vi "Test.vi"() -> ()   [LabVIEW 2010]
uses:
  Instance           5 12Saved   Test .vi
panel:
  out "Output ALG Msg Last Iter":string[][](table)=[["CODE", "PARAM"]]
  out "Output VOC Msg Last Iter":string[][](table)=[["CODE", "PARAM"]]
  out "Curr step ALG msg counter":i32
  out "Curr step VOC MSG counter":i32
  out "Params":string[](array[string])
  in  "STEP SIZE":i32(knob)=1 scale=1.0..10.0
  in  "Mode":bool
  in  "stop 2":bool
  in  "run":bool
  out "Result Input FOR VOC":u8[](array[numeric])
  out "output array":cluster{i32, "Value":string, i32}[](array[cluster])
  in  "Numeric":u8
  in  "Tab Control":T1(tab)=enum."Output ALG Info"
  out "ALG MSG queue":u8(slide) scale=0.0..5.0
  in  "send msg":bool
  in  "ALG MSG  PARAM":string
  in  "ALG MSG TYPE":string(combo)="0"
  in  "ALG MSG  CODE":string(combo)="1"
  out "VOC MSG queue":u8(slide) scale=0.0..5.0
  in  "send voc msg 2":bool
  in  "VOC MSG  PARAM":string
  in  "VOC MSG TYPE":string(combo)="0"
  in  "VOC MSG  CODE":string(combo)
  in  "VOC Last Interation MSG":i32(listbox)
  in  "VOC Param type":string(combo)
  out "Output Alg Ports":bool[](array[boolean])
  out "Output VOC Msg LOG":string[][](table)=[["CODE", "PARAM"]]
  out "VOC States":string[][](table)
  in  "ALG Param type":string(combo)
  in  "ALG Last Interation MSG":i32(listbox)
  out "Alg States":string[][](table)
  out "Input Alg Ports":bool[](array[boolean])
  out "Output Alg Msg":string[][](table)=[["CODE", "PARAM"]]
  in  "Save as new test":bool
  in  "Save changes in current test":bool
  in  "TEST":string="script_port: 8 /*index*/, 0 /* СЦЕНАРИЙ_ЛОГ_ВХОД_ПИТ_ВЕНТИЛЯТОРА*/ \r\nscript_port: 9 /*index*/, 0 /* СЦЕНАРИЙ_ЛОГ_ВХОД_ПИТ_РЕГ_Т*/ \r\nscript_port: 10 /*index*/, 0 /* СЦЕНАРИЙ_ЛОГ_ВХОД_НАС_ОХЛ*/ \r\nscript_port: 11 /*index*/, 0 /* СЦЕНАРИЙ_ЛОГ_ВХОД_ВАК_НАСОСА*/ \r\nscript_port: 12 /*index*/, 0 /* СЦЕНАРИЙ_ЛОГ_ВХОД_ЗАТВОР_ВАК*/ \r\nscript_port: 13 /*index*/, 0 /* СЦЕНАРИЙ_ЛОГ_ВХОД_САПУН*/ \r\nscript_port: 14 /*index*/, 0 /* СЦЕНАРИЙ_ЛОГ_ВХОД_УСТР_ПЛАВ_ПУСКА*/ \r\nscript_port: 15 /*index*/, 0 /* СЦЕНАРИЙ_ЛОГ_ВХОД_РЕГ_УР*/ \r\nscript_port: 16 /*index*/, 0 /* СЦЕНАРИЙ_ЛОГ_ВХОД_КОМПРЕССОР*/ \r\n\n\n\n\n\n\n\n"
  in  "Tests List":i32(listbox)
  out "voc code":i32[](array[numeric])=[-1, -1, -1, -1, -1, -1, -1, -1, -1, -1, -1, -1, -1, -1, -1, -1, -1, -1, -1, -1, -1, -1, -1, -1, -1, -1, -1, -1, -1, -1, -1, -1, -1, -1, -1, -1, -1, -1, -1, -1, -1, -1, -1, -1, -1, -1, -1, -1, -1, -1, -1, -1, -1, -1, -1, -1, -1, -1, -1, -1, -1, -1, -1, -1, -1, -1, -1, -1, -1, -1, -1, -1, -1, -1, -1, -1, -1, -1, -1, -1, -1, -1, -1, -1, -1, -1, -1, -1, -1, -1, -1, -1, -1, -1, -1, -1, -1, -1, -1, -1, -1, -1, -1, -1, -1, -1, -1, -1, -1, -1, -1, -1, -1, -1, -1, -1, -1, -1, -1, -1, -1, -1, -1, -1, -1, -1, -1, -1, -1, -1, -1, -1, -1, -1, -1, -1, -1, -1, -1, -1, -1, -1, -1, -1, -1, -1, -1, -1, -1, -1, -1, -1, -1, -1, -1, -1, -1, -1, -1, -1, -1, -1, -1, -1, -1, -1, -1, -1, -1, -1, -1, -1, -1, -1, -1, -1, -1, -1, -1, -1, -1, -1, -1, -1, -1, -1, -1, -1, -1, -1, -1, -1, -1, -1, -1, -1, -1, -1, -1, -1, -1, -1, -1, -1, -1, -1, -1, -1, -1, -1, -1, -1, -1, -1, -1, -1, -1, -1, -1, -1, -1, -1, -1, -1, -1, -1, -1, -1, -1, -1, -1, -1, -1, -1, -1, -1, -1, -1, -1, -1, -1, -1, -1, -1, -1, -1, -1, -1, -1, -1]
  out "VOC Out MSG Codes":string[](array[string])=["4", "5", "6", "7", "8", "9", "10", "11", "12", "13", "14", "15", "16", "17", "18", "19", "20", "21", "22", "23", "24", "25", "26", "27", "28", "29", "30", "31", "32", "33"]
  out "VOC Out MSG Names":string[](array[string])=["ПК_ТЕСТ_ГУИ_ОШИБКА_КОДА_КОМАНДЫ_ОТ_ГУИ", "ПК_ТЕСТ_ГУИ_ТЕМПЕРАТУРА_ВОДЫ_В_БАКЕ_ИЗМЕНИЛАСЬ", "ПК_ТЕСТ_ГУИ_ТЕМПЕРАТУРА_ВОДЫ_В_РУБАШКЕ_ИЗМЕНИЛАСЬ", "ПК_ТЕСТ_ГУИ_ТЕМПЕРАТУРА_НАСОСА_ИЗМЕНИЛАСЬ", "ПК_ТЕСТ_ГУИ_ВОДА_В_БАКЕ_ЗАКИПЕЛА", "ПК_ТЕСТ_ГУИ_ВОДА_В_БАКЕ_ЗАМЕРЗЛА", "ПК_ТЕСТ_ГУИ_ТЕМПЕРАТУРА_ВОДЫ_В_БАКЕ_СЛИШКОМ_ВЫСОКАЯ", "ПК_ТЕСТ_ГУИ_ТЕМПЕРАТУРА_ВОДЫ_В_БАКЕ_СЛИШКОМ_НИЗКАЯ", "ПК_ТЕСТ_ГУИ_ТЕМПЕРАТУРА_ОКУЖАЮЩЕЙ_СРЕДЫ_ИЗМЕНИЛАСЬ", "ПК_ТЕСТ_ГУИ_ТЕМПЕРАТУРА_ОКУЖАЮЩЕЙ_СРЕДЫ_СЛИШКОМ_ВЫСОКАЯ", "ПК_ТЕСТ_ГУИ_ТЕМПЕРАТУРА_ОКУЖАЮЩЕЙ_СРЕДЫ_СЛИШКОМ_НИЗКАЯ", "ПК_ТЕСТ_ГУИ_УРОВЕНЬ_ВОДЫ_НОРМ", "ПК_ТЕСТ_ГУИ_УРОВЕНЬ_ВОДЫ_MAX", "ПК_ТЕСТ_ГУИ_УРОВЕНЬ_ВОДЫ_MIN", "ПК_ТЕСТ_ГУИ_ДАВЛЕНИЕ_В_ТРУБЕ_СИДЕРОСТАТА_ИЗМЕНИЛОСЬ", "ПК_ТЕСТ_ГУИ_ДАВЛЕНИЕ_В_ТРУБЕ_СЛИШКОМ_ВЫСОКОЕ", "ПК_ТЕСТ_ГУИ_ДАВЛЕНИЕ_В_ТРУБЕ_СЛИШКОМ_НИЗКОЕ", "ПК_ТЕСТ_ГУИ_ДАВЛЕНИЕ_В_ПАТРУБКЕ_ИЗМЕНИЛОСЬ", "ПК_ТЕСТ_ГУИ_ДАВЛЕНИЕ_В_ПАТРУБКЕ_СЛИШКОМ_ВЫСОКОЕ", "ПК_ТЕСТ_ГУИ_ДАВЛЕНИЕ_В_ПАТРУБКЕ_СЛИШКОМ_НИЗКОЕ", "ПК_ТЕСТ_ГУИ_ДАВЛЕНИЕ_В_БАКЕ_КОМПРЕССОРА_ИЗМЕНИЛОСЬ", "ПК_ТЕСТ_ГУИ_ДАВЛЕНИЕ_В_КОМПРЕССОРЕ_СЛИШКОМ_НИЗКОЕ", "ПК_ТЕСТ_ГУИ_ОШИБКА_ПОПЫТКА_ОТКРЫТЬ_САПУН_ПРИ_ОТКРЫТОМ_ЗАТВОРЕ", "ПК_ТЕСТ_ГУИ_ОШИБКА_ПОПЫТКА_ОТКРЫТЬ_ЗАТВОР_ПРИ_ОТКРЫТОМ_САПУНЕ", "ПК_ТЕСТ_ГУИ_ОШИБКА_ДАВЛЕНИЕ_ПАТРУБКА_ВЫШЕ_ДАВЛЕНИЯ_ТРУБЫ", "ПК_ТЕСТ_ГУИ_ОШИБКА_ВКЛЮЧЕНИЕ_НАГРЕВА_ПРИ_НИЗКОМ_УРОВНЕ_ВОДЫ", "ПК_ТЕСТ_ГУИ_ПОПЫТКА_ЗАПУСКА_УСТР_ПЛАВ_ПУСКА_БЕЗ_ПИТАНИЯ", "ПК_ТЕСТ_ГУИ_ОШИБКА_ВКЛЮЧЕНИЕ_НАСОСА_ОХЛ_ПРИ_НИЗКОМ_УРОВНЕ_ВОДЫ", "ПК_ТЕСТ_ГУИ_ОШИБКА_ПЕРЕГРЕВ_ВАК_НАСОСА", "ПК_ТЕСТ_ГУИ_ОШИБКА_ОТКЛЮЧЕНИЕ_ПИТАНИЯ_ВКН_ПРИ_ЗАПУЩЕННОМ_ВКН"]
  out "output VOC array":cluster{i32, "Value":string, i32}[](array[cluster])=[{-1, "Value"="", 0}, {-1, "Value"="", 0}, {-1, "Value"="", 0}, {-1, "Value"="", 0}, {-1, "Value"="", 0}, {-1, "Value"="", 0}, {-1, "Value"="", 0}, {-1, "Value"="", 0}, {-1, "Value"="", 0}, {-1, "Value"="", 0}, {-1, "Value"="", 0}, {-1, "Value"="", 0}, {-1, "Value"="", 0}, {-1, "Value"="", 0}, {-1, "Value"="", 0}]
  out "input VOC array":cluster{i32, "Value":string, i32}[](array[cluster])
  out "AY states array":cluster{u32, u8}[](array[cluster])
  out "ALG output array":cluster{i32, "Value":string, i32}[](array[cluster])=[{-1, "Value"="", 0}, {-1, "Value"="", 0}, {-1, "Value"="", 0}, {-1, "Value"="", 0}, {-1, "Value"="", 0}]
  out "voc states array":cluster{u32, u8}[](array[cluster])
  out "ALG input array":cluster{i32, "Value":string, i32}[](array[cluster])
  out "VOC_STATES_SET":string[][](array[string])=[["Начало", " ", " ", " ", " ", " "], ["Начало", "НекорректноеСобытие", " ", " ", " ", " "], ["Начало", " ", " ", " ", " ", " "], ["Останов", " ", " ", " ", " ", " "], ["Начало", "Неисправность_вентилятора", " ", " ", " ", " "], ["Включение", "Вентилятор_ВКЛЮЧЕН", " ", " ", " ", " "], ["Выключение", "Вентилятор_ВЫКЛЮЧЕН", " ", " ", " ", " "], ["Начало", "Неисправность_Регулятора_Температуры", " ", " ", " ", " "], ["Включение", "Контроль_температуры_ВКЛЮЧЕН", "Временное_Отключение", "Кипение", " ", " "], ["Включение", "Контроль_температуры_ВЫКЛЮЧЕН", "СамопроизвольноеОхлаждение", "СамопроивольныйНагрев", "Замерзло", "ТепловоеРавновесие"], ["Начало", "Неисправность_регулятора_уровня", " ", " ", " ", " "], ["Включение", "Контроль_Рег_Уровня_ВКЛЮЧЕН", " ", " ", " ", " "], ["Включение", "Контроль_Рег_Уровня_ВЫКЛЮЧЕН", " ", " ", " ", " "], ["Начало", "Неисправность_Насоса_Охлаждения", " ", " ", " ", " "], ["Включение", "Контроль_Насоса_Охлажд_ВКЛЮЧЕН", "НАГРЕВ_НАСОСА_ОХЛАЖД_ВОДЫ", "ОХЛАЖД_НАСОСА_НАГРЕВ_ВОДЫ", "ТепловоеРавновесие", "Авария"], ["Включение", "Контроль_Насоса_Охлажд_ВЫКЛЮЧЕН", "САМОПРОИЗВ_ОХЛАЖД_НАСОСА", "САМОПРОИЗВ_НАГРЕВ_НАСОСА", "ТепловоеРавновесие", " "], ["Начало", "Неисправность_Сапуна", " ", " ", " ", " "], ["Открытие", "Сапун_ОТКРЫТ", " ", " ", " ", " "], ["Выключение", "Сапун_ЗАКРЫТ", " ", " ", " ", " "], ["Начало", "Неисправность_Затвора", " ", " ", " ", " "], ["Открытие", "Затвор_ОТКРЫТ", " ", " ", " ", " "], ["Закрытие", "Затвор_ЗАКРЫТ", " ", " ", " ", " "], ["Начало", "Неисправность_питания_насоса", " ", " ", " ", " "], ["Включение", "Питание_ПОДАНО", " ", " ", " ", " "], ["Выключение", "Задержка_перед_отключением", "Питание_ОТКЛЮЧЕНО", " ", " ", " "], ["Начало", "Неисправность_устр_плав_пуска", " ", " ", " ", " "], ["Включение", "Устр_Плав_Пуска_ЗАПУЩЕНО", "Вакуум", " ", " ", " "], ["Выключение", "Устр_Плав_Пуска_ОСТАНОВЛЕНО", " ", " ", " ", " "], ["Начало", "Исправность_Компрессора", "Неисправность_Компрессора", " ", " ", " "]]
  out "VOC_PROC":string[](array[string])=["Инициализация", "ЧтениеКольцевогоБуфера", "ЗАПОЛНЕНИЕ_ДОСТОВЕРНОСТЕЙ", "АварийноеЗавершениеРаботы", "УПРАВЛЕНИЕ_ВЕНТИЛЯТОРОМ", "ВКЛЮЧЕНИЕ_ВЕНТИЛЯТОРА", "ВЫКЛЮЧЕНИЕ_ВЕНТИЛЯТОРА", "УПРАВЛЕНИЕ_ТЕМПЕРАТУРОЙ", "ВКЛЮЧЕНИЕ_РЕГ_ТЕМПЕРАТУРЫ", "ВЫКЛЮЧЕНИЕ_РЕГ_ТЕМПЕРАТУРЫ", "УПРАВЛЕНИЕ_РЕГУЛЯТОРОМ_УР_ВОДЫ_В_БАКЕ", "ВКЛЮЧЕНИЕ_РЕГ_УРОВНЯ", "ВЫКЛЮЧЕНИЕ_РЕГ_УРОВНЯ", "УПРАВЛЕНИЕ_НАСОСОМ_ОХЛАЖДЕНИЯ", "ВКЛЮЧЕНИЕ_НАСОСА_ОХЛАЖД", "ВЫКЛЮЧЕНИЕ_НАСОСА_ОХЛАЖД", "УПРАВЛЕНИЕ_САПУНОМ", "ОТКРЫТИЕ_САПУНА", "ЗАКРЫТИЕ_САПУНА", "УПРАВЛЕНИЕ_ЗАТВОРОМ", "ОТКРЫТИЕ_ЗАТВОРА", "ЗАКРЫТИЕ_ЗАТВОРА", "УПРАВЛЕНИЕ_ПИТАНИЕМ_ВКН", "ПОДАЧА_ПИТАНИЯ_НА_ВКН", "ОТКЛЮЧЕНИЕ_ПИТАНИЯ_ВКН", "УПРАВЛЕНИЕ_УСТР_ПЛАВ_ПУСКА", "ЗАПУСК_УСТР_ПЛАВ_ПУСКА", "ОСТАНОВ_УСТР_ПЛАВ_ПУСКА", "УПРАВЛЕНИЕ_КОМПРЕССОРОМ"]
  out "Alg Out MSG Codes":string[](array[string])=["0", "1", "2", "3", "4", "5", "6", "7", "8", "9", "10", "11", "12", "13", "14", "15", "16", "41", "42", "43", "44", "45", "46", "47", "48", "49", "50", "51", "52", "53", "54", "55", "56", "57", "58", "59", "60", "61", "62", "63", "64", "65", "66", "67", "68", "69", "70", "71", "72", "73", "74", "75", "76", "77", "78", "79", "80", "81", "82", "83", "84", "85", "86", "87", "88", "89", "90", "91", "92", "93", "94", "95", "96", "97", "98", "99", "100", "101", "102", "103", "104", "105", "106", "107", "108", "109", "110", "111", "112", "113", "114", "115", "116", "117", "118", "119", "120", "121", "122", "123", "124", "125", "126", "127", "128", "129", "130", "135"]
  out "Alg Out MSG Names":string[](array[string])=["ПК_ГУИ_УРОВЕНЬ_ВОДЫ_В_БАКЕ_ОХЛАЖДЕНИЯ_НИЗКИЙ", "ПК_ГУИ_УРОВЕНЬ_ВОДЫ_В_БАКЕ_ОХЛАЖДЕНИЯ_ВЫСОКИЙ", "ПК_ГУИ_УРОВЕНЬ_ВОДЫ_В_БАКЕ_ОХЛАЖДЕНИЯ_В_НОРМЕ", "ПК_ГУИ_ОТКАЗ_ДАТЧИКОВ_УРОВНЯ", "ПК_ГУИ_ТЕМПЕРАТУРА_ВОДЫ_В_БАКЕ_ОХЛАЖДЕНИЯ_НИЗКАЯ", "ПК_ГУИ_ТЕМПЕРАТУРА_ВОДЫ_В_БАКЕ_ОХЛАЖДЕНИЯ_ВЫСОКАЯ", "ПК_ГУИ_ТЕМПЕРАТУРА_ВОДЫ_В_БАКЕ_ОХЛАЖДЕНИЯ_В_НОРМЕ", "ПК_ГУИ_ТЕМПЕРАТУРА_ВОДЫ_В_РУБАШКЕ_ОХЛАЖДЕНИЯ_НИЗКАЯ", "ПК_ГУИ_ТЕМПЕРАТУРА_ВОДЫ_В_РУБАШКЕ_ОХЛАЖДЕНИЯ_ВЫСОКАЯ", "ПК_ГУИ_ТЕМПЕРАТУРА_ВОДЫ_В_РУБАШКЕ_ОХЛАЖДЕНИЯ_В_НОРМЕ", "ПК_ГУИ_ДАВЛЕНИЕ_В_ВАКУУМНОЙ_ТРУБЕ_В_НОРМЕ", "ПК_ГУИ_ДАВЛЕНИЕ_В_ВАКУУМНОЙ_ТРУБЕ_ВНЕ_НОРМЫ", "ПК_ГУИ_СКОРОСТЬ_ОТКАЧКИ_В_НОРМЕ", "ПК_ГУИ_СКОРОСТЬ_ОТКАЧКИ_НИЖЕ_НОРМЫ", "ПК_ГУИ_ДАВЛЕНИЕ_В_БАКЕ_КОМПРЕССОРА_В_НОРМЕ", "ПК_ГУИ_ДАВЛЕНИЕ_В_БАКЕ_КОМПРЕССОРА_ВЫШЕ_НОРМЫ", "ПК_ГУИ_ДАВЛЕНИЕ_В_БАКЕ_КОМПРЕССОРА_НИЖЕ_НОРМЫ", "ПК_ГУИ_ОТКАЗ_ОТКРЫТИЯ_ЗАТВОРА_ВАКУУМНОГО", "ПК_ГУИ_ОТКАЗ_ЗАКРЫТИЯ_ЗАТВОРА_ВАКУУМНОГО", "ПК_ГУИ_ОТКАЗ_ОТКРЫТИЯ_САПУНА", "ПК_ГУИ_ОТКАЗ_ЗАКРЫТИЯ_САПУНА", "ПК_ГУИ_ОТКАЗ_ВКЛЮЧЕНИЯ_ВЕНТИЛЯТОРА", "ПК_ГУИ_ОТКАЗ_ВЫКЛЮЧЕНИЯ_ВЕНТИЛЯТОРА", "ПК_ГУИ_ОТКАЗ_ВКЛЮЧЕНИЯ_УСТР_ПЛАВ_ПУСКА", "ПК_ГУИ_ОТКАЗ_ВЫКЛЮЧЕНИЯ_УСТР_ПЛАВ_ПУСКА", "ПК_ГУИ_ОТКАЗ_ВКЛЮЧЕНИЯ_РЕГУЛЯТОРА_ТЕМПЕРАТУРЫ", "ПК_ГУИ_ОТКАЗ_ВЫКЛЮЧЕНИЯ_РЕГУЛЯТОРА_ТЕМПЕРАТУРЫ", "ПК_ГУИ_ОТКАЗ_ВКЛЮЧЕНИЯ_РЕГУЛЯТОРА_УРОВНЯ", "ПК_ГУИ_ОТКАЗ_ВЫКЛЮЧЕНИЯ_РЕГУЛЯТОРА_УРОВНЯ", "ПК_ГУИ_ОТКАЗ_ВКЛЮЧЕНИЯ_НАСОСА_ОХЛАЖДЕНИЯ", "ПК_ГУИ_ОТКАЗ_ВЫКЛЮЧЕНИЯ_НАСОСА_ОХЛАЖДЕНИЯ", "ПК_ГУИ_ИДЕТ_ВАКУУМИРОВАНИЕ_ОТКАЗ_ВЫПОЛНЕНИЯ_КОМАНДЫ", "ПК_ГУИ_НЕТ_УСЛОВИЙ_ДЛЯ_ВЫПОЛНЕНИЯ_КОМАНДЫ", "ПК_ГУИ_УРОВЕНЬ_ВОДЫ_В_БАКЕ_ОХЛАЖДЕНИЯ_ВНЕ_НОРМЫ_ОТКАЗ_ВЫПОЛНЕНИ", "ПК_ГУИ_ОТРИЦАТЕЛЬНАЯ_ТЕМПЕРАТУРА_ВОДЫ_ОТКАЗ_ВЫПОЛНЕНИЯ_КОМАНДЫ", "ПК_ГУИ_ДАВЛЕНИЕ_В_ПАТРУБКЕ_НЕ_УМЕНЬШАЕТСЯ", "ПК_ГУИ_ДАВЛЕНИЕ_В_ВАК_ТРУБЕ_НЕ_УМЕНЬШАЕТСЯ", "ПК_ГУИ_ВАКУУМИРОВАНИЕ_УСПЕШНО_ЗАВЕРШЕНО", "ПК_ГУИ_ОТКАЗ_ВКЛЮЧЕНИЯ_ПИТАНИЯ_ВАКУУМНОГО_НАСОСА", "ПК_ГУИ_ОТКАЗ_ВЫКЛЮЧЕНИЯ_ПИТАНИЯ_ВАКУУМНОГО_НАСОСА", "ПК_ГУИ_АВАРИЯ_НЕДОСТОВЕРНЫЕ_ДАННЫЕ_ОБОРУДОВАНИЯ_ВАК_СИСТЕМЫ", "ПК_ГУИ_ВЕНТИЛЯТОР_ВКЛЮЧЕН", "ПК_ГУИ_ВЕНТИЛЯТОР_ВЫКЛЮЧЕН", "ПК_ГУИ_СПОНТАННОЕ_ВЫКЛЮЧЕНИЕ_ВЕНТИЛЯТОРА", "ПК_ГУИ_СПОНТАННОЕ_ВКЛЮЧЕНИЕ_ВЕНТИЛЯТОРА", "ПК_ГУИ_ЗАТВОР_ВАКУУМНЫЙ_ОТКРЫТ", "ПК_ГУИ_ЗАТВОР_ВАКУУМНЫЙ_ЗАКРЫТ", "ПК_ГУИ_СРЕДНЕЕ_СОСТОЯНИЕ_ЗАТВОРА_ВАКУУМНОГО", "ПК_ГУИ_СОСТОЯНИЕ_ОШИБКИ_ЗАТВОРА_ВАКУУМНОГО", "ПК_ГУИ_СПОНТАННОЕ_ОТКРЫТИЕ_ЗАТ_ВАКУУМНОГО", "ПК_ГУИ_СПОНТАННОЕ_ЗАКРЫТИЕ_ЗАТ_ВАКУУМНОГО", "ПК_ГУИ_САПУН_ОТКРЫТ", "ПК_ГУИ_САПУН_ЗАКРЫТ", "ПК_ГУИ_СПОНТАННОЕ_ОТКРЫТИЕ_САПУНА", "ПК_ГУИ_СПОНТАННОЕ_ЗАКРЫТИЕ_САПУНА", "ПК_ГУИ_ПИТАНИЕ_ВАКУУМНОГО_НАСОСА_ВКЛЮЧЕНО", "ПК_ГУИ_ПИТАНИЕ_ВАКУУМНОГО_НАСОСА_ВЫКЛЮЧЕНО", "ПК_ГУИ_СПОНТАННОЕ_ВКЛЮЧЕНИЕ_ВАКУУМНОГО_НАСОСА", "ПК_ГУИ_СПОНТАННОЕ_ВЫКЛЮЧЕНИЕ_ВАКУУМНОГО_НАСОСА", "ПК_ГУИ_ПИТАНИЕ_РЕГУЛЯТОРА_ТЕМПЕРАТУРЫ_ВКЛЮЧЕНО", "ПК_ГУИ_ПИТАНИЕ_РЕГУЛЯТОРА_ТЕМПЕРАТУРЫ_ВЫКЛЮЧЕНО", "ПК_ГУИ_СПОНТАННОЕ_ВКЛЮЧЕНИЕ_РЕГУЛЯТОРА_ТЕМПЕРАТУРЫ", "ПК_ГУИ_СПОНТАННОЕ_ВЫКЛЮЧЕНИЕ_РЕГУЛЯТОРА_ТЕМПЕРАТУРЫ", "ПК_ГУИ_ПИТАНИЕ_РЕГУЛЯТОРА_УРОВНЯ_ВКЛЮЧЕНО", "ПК_ГУИ_ПИТАНИЕ_РЕГУЛЯТОРА_УРОВНЯ_ВЫКЛЮЧЕНО", "ПК_ГУИ_СПОНТАННОЕ_ВКЛЮЧЕНИЕ_РЕГУЛЯТОРА_УРОВНЯ", "ПК_ГУИ_СПОНТАННОЕ_ВЫКЛЮЧЕНИЕ_РЕГУЛЯТОРА_УРОВНЯ", "ПК_ГУИ_ПИТАНИЕ_НАСОСА_ОХЛАЖДЕНИЯ_ВКЛЮЧЕНО", "ПК_ГУИ_ПИТАНИЕ_НАСОСА_ОХЛАЖДЕНИЯ_ВЫКЛЮЧЕНО", "ПК_ГУИ_СПОНТАННОЕ_ВКЛЮЧЕНИЕ_НАСОСА_ОХЛАЖДЕНИЯ", "ПК_ГУИ_СПОНТАННОЕ_ВЫКЛЮЧЕНИЕ_НАСОСА_ОХЛАЖДЕНИЯ", "ПК_ГУИ_УСТРОЙСТВО_ПЛАВНОГО_ПУСКА_ВКЛЮЧЕНО", "ПК_ГУИ_УСТРОЙСТВО_ПЛАВНОГО_ПУСКА_ВЫКЛЮЧЕНО", "ПК_ГУИ_СПОНТАННОЕ_ВКЛЮЧЕНИЕ_УСТРОЙСТВА_ПЛАВНОГО_ПУСКА", "ПК_ГУИ_СПОНТАННОЕ_ВЫКЛЮЧЕНИЕ_УСТРОЙСТВА_ПЛАВНОГО_ПУСКА", "ПК_ГУИ_ОТКАЗ_ВАКУУМИРОВАНИЯ", "ПК_ГУИ_ОТКАЗ_ВКЛЮЧЕНИЯ_ВАКУУМНОЙ_ПОДСИСТЕМЫ", "ПК_ГУИ_ОТКАЗ_ВЫКЛЮЧЕНИЯ_ВАКУУМНОЙ_ПОДСИСТЕМЫ", "ПК_ГУИ_ЕСТЬ_ДОСТОВЕРНОСТЬ_КОНТРОЛЯ_ОТКРЫТИЯ_ЗАТВОРА_ВАКУУМНОГО", "ПК_ГУИ_НЕТ_ДОСТОВЕРНОСТИ_КОНТРОЛЯ_ОТКРЫТИЯ_ЗАТВОРА_ВАКУУМНОГО", "ПК_ГУИ_ЕСТЬ_ДОСТОВЕРНОСТЬ_КОНТРОЛЯ_ЗАКРЫТИЯ_ЗАТВОРА_ВАКУУМНОГО", "ПК_ГУИ_НЕТ_ДОСТОВЕРНОСТИ_КОНТРОЛЯ_ЗАКРЫТИЯ_ЗАТВОРА_ВАКУУМНОГО", "ПК_ГУИ_ЕСТЬ_ДОСТОВЕРНОСТЬ_КОНТРОЛЯ_САПУНА", "ПК_ГУИ_НЕТ_ДОСТОВЕРНОСТИ_КОНТРОЛЯ_САПУНА", "ПК_ГУИ_ЕСТЬ_ДОСТОВЕРНОСТЬ_КОНТРОЛЯ_УСТР_ПЛАВ_ПУСКА", "ПК_ГУИ_НЕТ_ДОСТОВЕРНОСТИ_КОНТРОЛЯ_УСТР_ПЛАВ_ПУСКА", "ПК_ГУИ_ЕСТЬ_ДОСТОВЕРНОСТЬ_КОНТРОЛЯ_ПИТ_ВАК_НАСОСА", "ПК_ГУИ_НЕТ_ДОСТОВЕРНОСТИ_КОНТРОЛЯ_ПИТ_ВАК_НАСОСА", "ПК_ГУИ_ЕСТЬ_ДОСТОВЕРНОСТЬ_КОНТРОЛЯ_ПИТ_ВЕНТИЛЯТОРА", "ПК_ГУИ_НЕТ_ДОСТОВЕРНОСТИ_КОНТРОЛЯ_ПИТ_ВЕНТИЛЯТОРА", "ПК_ГУИ_ЕСТЬ_ДОСТОВЕРНОСТЬ_РЕГ_ТЕМПЕРАТУРЫ", "ПК_ГУИ_НЕТ_ДОСТОВЕРНОСТИ_КОНТРОЛЯ_ПИТ_РЕГ_ТЕМПЕРАТУРЫ", "ПК_ГУИ_ЕСТЬ_ДОСТОВЕРНОСТЬ_РЕГ_УРОВНЯ", "ПК_ГУИ_НЕТ_ДОСТОВЕРНОСТИ_КОНТРОЛЯ_ПИТ_РЕГ_УРОВНЯ", "ПК_ГУИ_ЕСТЬ_ДОСТОВЕРНОСТЬ_МИНИМ_УР_ВОДЫ", "ПК_ГУИ_НЕТ_ДОСТОВЕРНОСТИ_МИНИМ_УР_ВОДЫ", "ПК_ГУИ_ЕСТЬ_ДОСТОВЕРНОСТЬ_МАКСИМ_УР_ВОДЫ", "ПК_ГУИ_НЕТ_ДОСТОВЕРНОСТИ_МАКСИМ_УР_ВОДЫ", "ПК_ГУИ_ЕСТЬ_ДОСТОВЕРНОСТЬ_КОНТРОЛЯ_ПИТ_НАСОСА_ОХЛ", "ПК_ГУИ_НЕТ_ДОСТОВЕРНОСТИ_КОНТРОЛЯ_ПИТ_НАСОСА_ОХЛ", "ПК_ГУИ_ВАКУУМИРОВАНИЕ_ТРУБЫ_ВКЛЮЧЕНО", "ПК_ГУИ_ВАКУУМИРОВАНИЕ_ТРУБЫ_ВЫКЛЮЧЕНО", "ПК_ГУИ_ФП_P_ВбакеКомпрессора", "ПК_ГУИ_ФП_P_Впатрубке", "ПК_ГУИ_ФП_T_Врубашке", "ПК_ГУИ_ФП_T_Вбаке", "ПК_ГУИ_ФП_P_ВтрубеСидер", "ПК_ГУИ_ОШИБКА_КОДА_КОМАНДЫ_ОТ_ГУИ"]
  out "AY_STATES_SET":string[][](array[string])=[["Начало", "ВосстановлениеУправления", "НачалоРаботы", " ", " ", " ", " ", " ", " ", " ", " ", " ", " ", " ", " ", " ", " ", " ", " ", " ", " ", " ", " ", " ", " ", " ", " ", " ", " ", " "], ["Начало", " ", " ", " ", " ", " ", " ", " ", " ", " ", " ", " ", " ", " ", " ", " ", " ", " ", " ", " ", " ", " ", " ", " ", " ", " ", " ", " ", " ", " "], ["Начало", "ОстановПроцессов", "СообК_ГУИ_НЕТ_ДОСТОВЕРНОСТИ", "НарушениеСвязи", " ", " ", " ", " ", " ", " ", " ", " ", " ", " ", " ", " ", " ", " ", " ", " ", " ", " ", " ", " ", " ", " ", " ", " ", " ", " "], ["Начало", "СменаСостоянияВКЛ", "СменаСостоянияВЫКЛ", "ТрафикПауза", "НарушениеСвязи", " ", " ", " ", " ", " ", " ", " ", " ", " ", " ", " ", " ", " ", " ", " ", " ", " ", " ", " ", " ", " ", " ", " ", " ", " "], ["Начало", "СообК_ГУИ_ЕСТЬ_ДОСТОВЕРНОСТЬ", "ОжиданиеНедостоверности", "СообК_ГУИ_НЕТ_ДОСТОВЕРНОСТИ", "ОжиданиеЕстьДостоверность", "НарушениеСвязи", " ", " ", " ", " ", " ", " ", " ", " ", " ", " ", " ", " ", " ", " ", " ", " ", " ", " ", " ", " ", " ", " ", " ", " "], ["Начало", "СообК_ГУИ_ЕСТЬ_ДОСТОВЕРНОСТЬ", "ОжиданиеНедостоверности", "СообК_ГУИ_НЕТ_ДОСТОВЕРНОСТИ", "ОжиданиеЕстьДостоверность", "НарушениеСвязи", " ", " ", " ", " ", " ", " ", " ", " ", " ", " ", " ", " ", " ", " ", " ", " ", " ", " ", " ", " ", " ", " ", " ", " "], ["Начало", "СообК_ГУИ_ЕСТЬ_ДОСТОВЕРНОСТЬ", "ОжиданиеНедостоверности", "СообК_ГУИ_НЕТ_ДОСТОВЕРНОСТИ", "ОжиданиеЕстьДостоверность", "НарушениеСвязи", " ", " ", " ", " ", " ", " ", " ", " ", " ", " ", " ", " ", " ", " ", " ", " ", " ", " ", " ", " ", " ", " ", " ", " "], ["Начало", "СообК_ГУИ_ЕСТЬ_ДОСТОВЕРНОСТЬ", "ОжиданиеНедостоверности", "СообК_ГУИ_НЕТ_ДОСТОВЕРНОСТИ", "ОжиданиеЕстьДостоверность", "НарушениеСвязи", " ", " ", " ", " ", " ", " ", " ", " ", " ", " ", " ", " ", " ", " ", " ", " ", " ", " ", " ", " ", " ", " ", " ", " "], ["Начало", "СообК_ГУИ_ЕСТЬ_ДОСТОВЕРНОСТЬ", "ОжиданиеНедостоверности", "СообК_ГУИ_НЕТ_ДОСТОВЕРНОСТИ", "ОжиданиеЕстьДостоверность", "НарушениеСвязи", " ", " ", " ", " ", " ", " ", " ", " ", " ", " ", " ", " ", " ", " ", " ", " ", " ", " ", " ", " ", " ", " ", " ", " "], ["Начало", "СообК_ГУИ_ЕСТЬ_ДОСТОВЕРНОСТЬ", "ОжиданиеНедостоверности", "СообК_ГУИ_НЕТ_ДОСТОВЕРНОСТИ", "ОжиданиеЕстьДостоверность", "НарушениеСвязи", " ", " ", " ", " ", " ", " ", " ", " ", " ", " ", " ", " ", " ", " ", " ", " ", " ", " ", " ", " ", " ", " ", " ", " "], ["Начало", "СообК_ГУИ_ЕСТЬ_ДОСТОВЕРНОСТЬ", "ОжиданиеНедостоверности", "СообК_ГУИ_НЕТ_ДОСТОВЕРНОСТИ", "ОжиданиеЕстьДостоверность", "НарушениеСвязи", " ", " ", " ", " ", " ", " ", " ", " ", " ", " ", " ", " ", " ", " ", " ", " ", " ", " ", " ", " ", " ", " ", " ", " "], ["Начало", "СообК_ГУИ_ЕСТЬ_ДОСТОВЕРНОСТЬ", "ОжиданиеНедостоверности", "СообК_ГУИ_НЕТ_ДОСТОВЕРНОСТИ", "ОжиданиеЕстьДостоверность", "НарушениеСвязи", " ", " ", " ", " ", " ", " ", " ", " ", " ", " ", " ", " ", " ", " ", " ", " ", " ", " ", " ", " ", " ", " ", " ", " "], ["Начало", "СообК_ГУИ_ЕСТЬ_ДОСТОВЕРНОСТЬ", "ОжиданиеНедостоверности", "СообК_ГУИ_НЕТ_ДОСТОВЕРНОСТИ", "ОжиданиеЕстьДостоверность", "НарушениеСвязи", " ", " ", " ", " ", " ", " ", " ", " ", " ", " ", " ", " ", " ", " ", " ", " ", " ", " ", " ", " ", " ", " ", " ", " "], ["Начало", "СообК_ГУИ_ЕСТЬ_ДОСТОВЕРНОСТЬ", "ОжиданиеНедостоверности", "СообК_ГУИ_НЕТ_ДОСТОВЕРНОСТИ", "ОжиданиеЕстьДостоверность", "НарушениеСвязи", " ", " ", " ", " ", " ", " ", " ", " ", " ", " ", " ", " ", " ", " ", " ", " ", " ", " ", " ", " ", " ", " ", " ", " "], ["Начало", "СообК_ГУИ_ЕСТЬ_ДОСТОВЕРНОСТЬ", "ОжиданиеНедостоверности", "СообК_ГУИ_НЕТ_ДОСТОВЕРНОСТИ", "ОжиданиеЕстьДостоверность", "НарушениеСвязи", " ", " ", " ", " ", " ", " ", " ", " ", " ", " ", " ", " ", " ", " ", " ", " ", " ", " ", " ", " ", " ", " ", " ", " "], ["Начало", " ", " ", " ", " ", " ", " ", " ", " ", " ", " ", " ", " ", " ", " ", " ", " ", " ", " ", " ", " ", " ", " ", " ", " ", " ", " ", " ", " ", " "], ["Начало", " ", " ", " ", " ", " ", " ", " ", " ", " ", " ", " ", " ", " ", " ", " ", " ", " ", " ", " ", " ", " ", " ", " ", " ", " ", " ", " ", " ", " "], ["Начало", "КонтрольВыполненияК", "КонтрольИзмененияНП", "НекорректноеСобытие", "НарушениеСвязи", " ", " ", " ", " ", " ", " ", " ", " ", " ", " ", " ", " ", " ", " ", " ", " ", " ", " ", " ", " ", " ", " ", " ", " ", " "], ["Анализ", "ПодтверждениеИзмененияНП", "НекорректноеСобытие", "НарушениеСвязи", " ", " ", " ", " ", " ", " ", " ", " ", " ", " ", " ", " ", " ", " ", " ", " ", " ", " ", " ", " ", " ", " ", " ", " ", " ", " "], ["Анализ", "НекорректноеСобытие", "ПередачаСообщенияСПараметромГУИ", "НарушениеСвязи", " ", " ", " ", " ", " ", " ", " ", " ", " ", " ", " ", " ", " ", " ", " ", " ", " ", " ", " ", " ", " ", " ", " ", " ", " ", " "], ["Начало", "КонтрольИзменения", "СообщОбИзменении", "ТрафикПауза", "НарушениеСвязи", " ", " ", " ", " ", " ", " ", " ", " ", " ", " ", " ", " ", " ", " ", " ", " ", " ", " ", " ", " ", " ", " ", " ", " ", " "], ["Начало", "КонтрольИзменения", "СообщОбИзменении", "ТрафикПауза", "НарушениеСвязи", " ", " ", " ", " ", " ", " ", " ", " ", " ", " ", " ", " ", " ", " ", " ", " ", " ", " ", " ", " ", " ", " ", " ", " ", " "], ["Начало", "КонтрольИзменения", "СообщОбИзменении", "ТрафикПауза", "НарушениеСвязи", " ", " ", " ", " ", " ", " ", " ", " ", " ", " ", " ", " ", " ", " ", " ", " ", " ", " ", " ", " ", " ", " ", " ", " ", " "], ["Начало", "КонтрольИзменения", "СообщОбИзменении", "ТрафикПауза", "НарушениеСвязи", " ", " ", " ", " ", " ", " ", " ", " ", " ", " ", " ", " ", " ", " ", " ", " ", " ", " ", " ", " ", " ", " ", " ", " ", " "], ["Начало", "КонтрольИзменения", "СообщОбИзменении", "ТрафикПауза", "НарушениеСвязи", " ", " ", " ", " ", " ", " ", " ", " ", " ", " ", " ", " ", " ", " ", " ", " ", " ", " ", " ", " ", " ", " ", " ", " ", " "], ["Начало", "АнализОткачки", " ", " ", " ", " ", " ", " ", " ", " ", " ", " ", " ", " ", " ", " ", " ", " ", " ", " ", " ", " ", " ", " ", " ", " ", " ", " ", " ", " "], ["Начало", "ДавлениеНормальное", "ДавлениеВысокое", "Задержка", "НарушениеСвязи", " ", " ", " ", " ", " ", " ", " ", " ", " ", " ", " ", " ", " ", " ", " ", " ", " ", " ", " ", " ", " ", " ", " ", " ", " "], ["Начало", "НизкийУровеньВоды", "ВысокийУровеньВоды", "УровеньВодыВнорме", "Задержка", "НарушениеСвязи", " ", " ", " ", " ", " ", " ", " ", " ", " ", " ", " ", " ", " ", " ", " ", " ", " ", " ", " ", " ", " ", " ", " ", " "], ["Начало", "НизкаяТемператураВоды", "ВысокаяТемператураВоды", "ТемператураВнорме", "Задержка", "НарушениеСвязи", " ", " ", " ", " ", " ", " ", " ", " ", " ", " ", " ", " ", " ", " ", " ", " ", " ", " ", " ", " ", " ", " ", " ", " "], ["Начало", "НизкаяТемператураВоды", "ВысокаяТемператураВоды", "ТемператураВнорме", "Задержка", "НарушениеСвязи", " ", " ", " ", " ", " ", " ", " ", " ", " ", " ", " ", " ", " ", " ", " ", " ", " ", " ", " ", " ", " ", " ", " ", " "], ["Начало", "НизкоеДавление", "ДавлениеВнорме", "Задержка", "НарушениеСвязи", " ", " ", " ", " ", " ", " ", " ", " ", " ", " ", " ", " ", " ", " ", " ", " ", " ", " ", " ", " ", " ", " ", " ", " ", " "], ["Начало", "КонтрольВключения", "ПередачаСообщения", "Ошибка", "НарушениеСвязи", " ", " ", " ", " ", " ", " ", " ", " ", " ", " ", " ", " ", " ", " ", " ", " ", " ", " ", " ", " ", " ", " ", " ", " ", " "], ["Начало", "КонтрольВыключения", "ПередачаСообщения", "Ошибка", "НарушениеСвязи", " ", " ", " ", " ", " ", " ", " ", " ", " ", " ", " ", " ", " ", " ", " ", " ", " ", " ", " ", " ", " ", " ", " ", " ", " "], ["Начало", "СменаСостоянияВКЛ", "СменаСостоянияВЫКЛ", "НарушениеСвязи", " ", " ", " ", " ", " ", " ", " ", " ", " ", " ", " ", " ", " ", " ", " ", " ", " ", " ", " ", " ", " ", " ", " ", " ", " ", " "], ["Контроль", "Ошибка", "НарушениеСвязи", " ", " ", " ", " ", " ", " ", " ", " ", " ", " ", " ", " ", " ", " ", " ", " ", " ", " ", " ", " ", " ", " ", " ", " ", " ", " ", " "], ["Контроль", "Ошибка", "НарушениеСвязи", " ", " ", " ", " ", " ", " ", " ", " ", " ", " ", " ", " ", " ", " ", " ", " ", " ", " ", " ", " ", " ", " ", " ", " ", " ", " ", " "], ["Начало", "СменаСостоянияСреднего", "СменаСостоянияЗакрытия", "СменаСостоянияОткрытия", "СменаСостоянияОшибки", "НарушениеСвязи", " ", " ", " ", " ", " ", " ", " ", " ", " ", " ", " ", " ", " ", " ", " ", " ", " ", " ", " ", " ", " ", " ", " ", " "], ["Начало", "Контроль", "ПередачаСообщения", "Ошибка", "НарушениеСвязи", " ", " ", " ", " ", " ", " ", " ", " ", " ", " ", " ", " ", " ", " ", " ", " ", " ", " ", " ", " ", " ", " ", " ", " ", " "], ["Начало", "Контроль", "ПередачаСообщения", "Ошибка", "НарушениеСвязи", " ", " ", " ", " ", " ", " ", " ", " ", " ", " ", " ", " ", " ", " ", " ", " ", " ", " ", " ", " ", " ", " ", " ", " ", " "], ["КонтрольЗакрытия", "Ошибка", "НарушениеСвязи", " ", " ", " ", " ", " ", " ", " ", " ", " ", " ", " ", " ", " ", " ", " ", " ", " ", " ", " ", " ", " ", " ", " ", " ", " ", " ", " "], ["Контроль", "Ошибка", "НарушениеСвязи", " ", " ", " ", " ", " ", " ", " ", " ", " ", " ", " ", " ", " ", " ", " ", " ", " ", " ", " ", " ", " ", " ", " ", " ", " ", " ", " "], ["Начало", "КонтрольОткрытия", "ПередачаСообщения", "Ошибка", "НарушениеСвязи", " ", " ", " ", " ", " ", " ", " ", " ", " ", " ", " ", " ", " ", " ", " ", " ", " ", " ", " ", " ", " ", " ", " ", " ", " "], ["Начало", "КонтрольЗакрытия", "ПередачаСообщения", "Ошибка", "НарушениеСвязи", " ", " ", " ", " ", " ", " ", " ", " ", " ", " ", " ", " ", " ", " ", " ", " ", " ", " ", " ", " ", " ", " ", " ", " ", " "], ["Начало", "СменаСостоянияВКЛ", "СменаСостоянияВЫКЛ", "НарушениеСвязи", " ", " ", " ", " ", " ", " ", " ", " ", " ", " ", " ", " ", " ", " ", " ", " ", " ", " ", " ", " ", " ", " ", " ", " ", " ", " "], ["КонтрольЗакрытия", "Ошибка", "НарушениеСвязи", " ", " ", " ", " ", " ", " ", " ", " ", " ", " ", " ", " ", " ", " ", " ", " ", " ", " ", " ", " ", " ", " ", " ", " ", " ", " ", " "], ["Контроль", "Ошибка", "НарушениеСвязи", " ", " ", " ", " ", " ", " ", " ", " ", " ", " ", " ", " ", " ", " ", " ", " ", " ", " ", " ", " ", " ", " ", " ", " ", " ", " ", " "], ["Начало", "КонтрольВключения", "ПередачаСообщения", "Ошибка", "НарушениеСвязи", " ", " ", " ", " ", " ", " ", " ", " ", " ", " ", " ", " ", " ", " ", " ", " ", " ", " ", " ", " ", " ", " ", " ", " ", " "], ["Начало", "КонтрольВыключения", "Ошибка", "НарушениеСвязи", "ПередачаСообщения", " ", " ", " ", " ", " ", " ", " ", " ", " ", " ", " ", " ", " ", " ", " ", " ", " ", " ", " ", " ", " ", " ", " ", " ", " "], ["Начало", "СменаСостоянияВКЛ", "СменаСостоянияВЫКЛ", "НарушениеСвязи", " ", " ", " ", " ", " ", " ", " ", " ", " ", " ", " ", " ", " ", " ", " ", " ", " ", " ", " ", " ", " ", " ", " ", " ", " ", " "], ["Контроль", "Ошибка", "НарушениеСвязи", " ", " ", " ", " ", " ", " ", " ", " ", " ", " ", " ", " ", " ", " ", " ", " ", " ", " ", " ", " ", " ", " ", " ", " ", " ", " ", " "], ["Контроль", "Ошибка", "НарушениеСвязи", " ", " ", " ", " ", " ", " ", " ", " ", " ", " ", " ", " ", " ", " ", " ", " ", " ", " ", " ", " ", " ", " ", " ", " ", " ", " ", " "], ["Начало", "КонтрольВключения", "ПередачаСообщения", "Ошибка", "НарушениеСвязи", " ", " ", " ", " ", " ", " ", " ", " ", " ", " ", " ", " ", " ", " ", " ", " ", " ", " ", " ", " ", " ", " ", " ", " ", " "], ["Начало", "КонтрольВыключения", "ПередачаСообщения", "Ошибка", "НарушениеСвязи", " ", " ", " ", " ", " ", " ", " ", " ", " ", " ", " ", " ", " ", " ", " ", " ", " ", " ", " ", " ", " ", " ", " ", " ", " "], ["Начало", "СменаСостоянияВКЛ", "СменаСостоянияВЫКЛ", "НарушениеСвязи", " ", " ", " ", " ", " ", " ", " ", " ", " ", " ", " ", " ", " ", " ", " ", " ", " ", " ", " ", " ", " ", " ", " ", " ", " ", " "], ["Контроль", "Ошибка", "НарушениеСвязи", " ", " ", " ", " ", " ", " ", " ", " ", " ", " ", " ", " ", " ", " ", " ", " ", " ", " ", " ", " ", " ", " ", " ", " ", " ", " ", " "], ["Контроль", "Ошибка", "НарушениеСвязи", " ", " ", " ", " ", " ", " ", " ", " ", " ", " ", " ", " ", " ", " ", " ", " ", " ", " ", " ", " ", " ", " ", " ", " ", " ", " ", " "], ["Начало", "Контроль", "ПередачаСообщения", "Ошибка", "НарушениеСвязи", " ", " ", " ", " ", " ", " ", " ", " ", " ", " ", " ", " ", " ", " ", " ", " ", " ", " ", " ", " ", " ", " ", " ", " ", " "], ["Начало", "Контроль", "ПередачаСообщения", "Ошибка", "НарушениеСвязи", " ", " ", " ", " ", " ", " ", " ", " ", " ", " ", " ", " ", " ", " ", " ", " ", " ", " ", " ", " ", " ", " ", " ", " ", " "], ["Начало", "СменаСостоянияВКЛ", "СменаСостоянияВЫКЛ", "НарушениеСвязи", " ", " ", " ", " ", " ", " ", " ", " ", " ", " ", " ", " ", " ", " ", " ", " ", " ", " ", " ", " ", " ", " ", " ", " ", " ", " "], ["Контроль", "Ошибка", "НарушениеСвязи", " ", " ", " ", " ", " ", " ", " ", " ", " ", " ", " ", " ", " ", " ", " ", " ", " ", " ", " ", " ", " ", " ", " ", " ", " ", " ", " "], ["Контроль", "Ошибка", "НарушениеСвязи", " ", " ", " ", " ", " ", " ", " ", " ", " ", " ", " ", " ", " ", " ", " ", " ", " ", " ", " ", " ", " ", " ", " ", " ", " ", " ", " "], ["Начало", "ВключениеПитания", "Контроль", "ПередачаСообщения", "Ошибка", "НарушениеСвязи", " ", " ", " ", " ", " ", " ", " ", " ", " ", " ", " ", " ", " ", " ", " ", " ", " ", " ", " ", " ", " ", " ", " ", " "], ["Начало", "Контроль", "ПередачаСообщения", "Ошибка", "НарушениеСвязи", " ", " ", " ", " ", " ", " ", " ", " ", " ", " ", " ", " ", " ", " ", " ", " ", " ", " ", " ", " ", " ", " ", " ", " ", " "], ["Начало", "СменаСостоянияВКЛ", "СменаСостоянияВЫКЛ", "НарушениеСвязи", " ", " ", " ", " ", " ", " ", " ", " ", " ", " ", " ", " ", " ", " ", " ", " ", " ", " ", " ", " ", " ", " ", " ", " ", " ", " "], ["Контроль", "Ошибка", "НарушениеСвязи", " ", " ", " ", " ", " ", " ", " ", " ", " ", " ", " ", " ", " ", " ", " ", " ", " ", " ", " ", " ", " ", " ", " ", " ", " ", " ", " "], ["Контроль", "Ошибка", "НарушениеСвязи", " ", " ", " ", " ", " ", " ", " ", " ", " ", " ", " ", " ", " ", " ", " ", " ", " ", " ", " ", " ", " ", " ", " ", " ", " ", " ", " "], ["Начало", "Контроль", "ПередачаСообщения", "Ошибка", "НарушениеСвязи", " ", " ", " ", " ", " ", " ", " ", " ", " ", " ", " ", " ", " ", " ", " ", " ", " ", " ", " ", " ", " ", " ", " ", " ", " "], ["Начало", "КонтрольВыключения", "ПередачаСообщения", "Ошибка", "НарушениеСвязи", " ", " ", " ", " ", " ", " ", " ", " ", " ", " ", " ", " ", " ", " ", " ", " ", " ", " ", " ", " ", " ", " ", " ", " ", " "], ["Начало", "СменаСостоянияВКЛ", "СменаСостоянияВЫКЛ", "НарушениеСвязи", " ", " ", " ", " ", " ", " ", " ", " ", " ", " ", " ", " ", " ", " ", " ", " ", " ", " ", " ", " ", " ", " ", " ", " ", " ", " "], ["Контроль", "Ошибка", "НарушениеСвязи", " ", " ", " ", " ", " ", " ", " ", " ", " ", " ", " ", " ", " ", " ", " ", " ", " ", " ", " ", " ", " ", " ", " ", " ", " ", " ", " "], ["Контроль", "Ошибка", "НарушениеСвязи", " ", " ", " ", " ", " ", " ", " ", " ", " ", " ", " ", " ", " ", " ", " ", " ", " ", " ", " ", " ", " ", " ", " ", " ", " ", " ", " "], ["Начало", "ПроверкаНеобходимостиВакуумирования", "ПередачаСообщения", "КонтрольВключенияВакПодсистемы", "ЗапоминаемДавлениеВвакуумнойТрубе", "КонтрольТемпературыРубашки", "КонтрольРаботыОборудования", "КонтрольДавления", "СообщениеОКонцеВакуумирования", "ПаузаНаРазвакуумированиеТрубы", "ПаузаНаОткачкуВвакуумнойТрубе", "ПроверкаУменьшенияДавленияВпатрубке", "ОткачкаОтсутствует", "ВыключениеВакуумнойПодсистемы", "СообщениеОбОтказеВакуумирования", "НарушениеСвязи", " ", " ", " ", " ", " ", " ", " ", " ", " ", " ", " ", " ", " ", " "], ["Начало", "ПередачаСообщения", "ВыключениеВакуумнойПодсистемы", "НарушениеСвязи", " ", " ", " ", " ", " ", " ", " ", " ", " ", " ", " ", " ", " ", " ", " ", " ", " ", " ", " ", " ", " ", " ", " ", " ", " ", " "], ["Начало", "ВключениеПитанияРегУровня", "КонтрольВключенияПитРегУр", "КонтрольГотовностиУровняВодыБО", "ВключениеРегТ", "КонтрольВключенияРегТ", "КонтрольПревышенияТемпературыВодыБО", "КонтрольГотовностиТемпературыВодыБО", "ВключаемВентилятор", "КонтрольВключенияВентилятора", "КонтрольВключенияПитанияНасосаОхлаждения", "КонтрольЗакрытияЗатвораВакуумного", "КонтрольОткрытияСапуна", "КонтрольТемпературыРубашки", "ПодачаПитанияНаВакуумныйНасос", "КонтрольПитанияВакуумногоНасоса", "ВключениеУстройстваПлавногоПуска", "КонтрольВлюченияПлавногоПуска", "ТаймаутПередЗакрытиемСапуна", "ЗакрытиеСапуна", "КонтрольЗакрытияСапуна", "ЗапоминаемДавлениеВпатрубке", "КонтрольДавления", "ПаузаНаОткачкуВпатрубке", "ПроверкаУменьшенияДавленияВпатрубке", "КонтрольОткрытияЗВ", "Ошибка", "ВыключениеПоОшибке", "СообщениеОбОтказеВакуумирования", "НарушениеСвязи"], ["Начало", "КонтрольЗакрытияЗатвораВакуумного", "КонтрольОткрытияСапуна", "ТаймаутПередВыключениемПитанияВакуумногоНасоса", "ВыключаемУППВакуумногоНасоса", "КонтрольВыключенияПитанияУППВакуумногоНасоса", "КонтрольВыключенияПитанияВакуумногоНасоса", "КонтрольВыключенияНасосаОхлаждения", "КонтрольВыключенияВентилятора", "СообщениеОбОтказеВыклВакСистемы", "НарушениеСвязи", " ", " ", " ", " ", " ", " ", " ", " ", " ", " ", " ", " ", " ", " ", " ", " ", " ", " ", " "]]
  out "AY_PROC":string[](array[string])=["Инициализация", "ОстановВсехПроцессовИстартПроцИнициализация", "КонтрольДостоверности", "КонтрольДостоверностиОткрытияЗатвораВакуумного", "КонтрольДостоверностиОткрЗатВакуумного", "КонтрольДостоверностиЗакрЗатВакуумного", "КонтрольДостоверностиСостоянияСапуна", "КонтрольДостоверностиСостоянияУстройстваПлавПуска", "КонтрольДостоверностиСостоянияПитанияВакуумногоНасоса", "КонтрольДостоверностиСостоянияПитанияВентилятора", "КонтрольДостоверностиСостоянияПитанияРегТемпературы", "КонтрольДостоверностиСостоянияПитанияРегУровня", "КонтрольДостоверностиУровняВодыМинимум", "КонтрольДостоверностиУровняВодыМаксимум", "КонтрольДостоверностиСостоянияПитанияНасОхлаждения", "ЧтениеФактПараметров_с_Датчиков", "РЕГУЛЯТОР_ТРАФИКА", "ЧтениеКольцевогоБуфера", "ОбработкаКомандИзмененияНП_от_ГУИ", "ОбработкаКомандУправления_от_ГУИ", "КонтрольИзменения_ФП_P_ВбакеКомпрессора", "КонтрольИзменения_ФП_P_Впатрубке", "КонтрольИзменения_ФП_T_Врубашке", "КонтрольИзменения_ФП_T_Вбаке", "КонтрольИзменения_ФП_P_ВтрубеСидер", "КонтрольВеличиныОткачкиВауумнойТрубыСидеростата", "КонтрольГотовностиВакуума_в_Вакуумной_Трубе", "КонтрольУровняВодыБакаОхлаждения", "КонтрольТемпературыВодыБакаОхлаждения", "КонтрольТемпературыРубашкиОхлаждения", "КонтрольДавленияВбакеКомпрессора", "ВКЛ_ПИТ_ВЕНТИЛЯТОР", "ВЫК_ПИТ_ВЕНТИЛЯТОР", "КонтрольСостоянияПитанияВентилятора", "КонтрольСпонтанногоВыключенияВентилятора", "КонтрольСпонтанногоВключенияВентилятора", "КонтрольСостоянияЗатвораВакуумного", "ОТКР_ЗАТВОР_ВАК", "ЗАКР_ЗАТВОР_ВАК", "КонтрольСпонтанногоЗакрытияЗатвораВакуумного", "КонтрольСпонтанногоОткрытияЗатвораВакуумного", "ОТКР_САПУН", "ЗАКР_САПУН", "КонтрольСостоянияПитанияСапуна", "КонтрольСпонтанногоЗакрытияСапуна", "КонтрольСпонтанногоОткрытияСапуна", "ВКЛ_ПИТ_ВАК_НАСОСА", "ВЫК_ПИТ_ВАК_НАСОСА", "КонтрольСостоянияПитанияВакуумногоНасоса", "КонтрольСпонтанногоВыключенияВакНасоса", "КонтрольСпонтанногоВключенияВакНасоса", "ВКЛ_ПИТ_РЕГ_Т", "ВЫК_ПИТ_РЕГ_Т", "КонтрольСостоянияПитанияРЕГ_Т", "КонтрольСпонтанногоВыключенияРЕГ_Т", "КонтрольСпонтанногоВключенияРЕГ_Т", "ВКЛ_ПИТ_РЕГ_УР", "ВЫК_ПИТ_РЕГ_УР", "КонтрольСостоянияПитанияРЕГ_УР", "КонтрольСпонтанногоВыключенияРЕГ_УР", "КонтрольСпонтанногоВключенияРЕГ_УР", "ВКЛ_ПИТ_НАС_ОХЛ", "ВЫК_ПИТ_НАС_ОХЛ", "КонтрольСостоянияПитанияНАС_ОХЛ", "КонтрольСпонтанногоВыключенияНасосаОхлаждения", "КонтрольСпонтанногоВключенияНасосаОхлаждения", "ВКЛ_УСТР_ПЛАВ_ПУСКА", "ВЫК_УСТР_ПЛАВ_ПУСКА", "КонтрольСостоянияПитанияПЛАВ_ПУСКА", "КонтрольСпонтанногоВыключенияПлавнПуска", "КонтрольСпонтанногоВключенияПлавнПуска", "ВКЛ_ВАКУУМИРОВАНИЕ_ТРУБЫ", "ВЫК_ВАКУУМИРОВАНИЕ_ТРУБЫ", "ВКЛ_ВАКУУМНУЮ_ПОДСИСТЕМУ", "ВЫК_ВАКУУМНУЮ_ПОДСИСТЕМУ"]
  out "Init  VOC INPUT":u8[](array[numeric])
  out "Alg Input":i32[](array[numeric])=[2, 2, 2, 2, 2, 2, 2, 2, 2, 2, 2]
  out "Alg Output":i32[](array[numeric])
  out "Init VOC output":u8[](array[numeric])
  in  "stop":bool
  # "STEP MODE"
  # "CONTINUOUS MODE"
  # "ALG MSG Generation"
  # "VOC MSG Generation"
  # "У_ПИТ_ВЕНТИЛЯТОРА"
  # "У_ПИТ_РЕГ_Т"
  # "У_ПИТ_НАС_ОХЛ"
  # "У_ПИТ_ВАК_НАСОСА"
  # "У_ЗАТВОР_ВАК"
  # "У_САПУН"
  # "У_УСТР_ПЛАВ_ПУСКА"
  # "У_ПИТ_РЕГ_УР"
  # "К_ОТКР_ЗАТВОР_ВАК"
  # "К_ЗАКР_ЗАТВОР_ВАК"
  # "К_САПУН"
  # "К_УСТР_ПЛАВ_ПУСКА"
  # "К_ПИТ_ВАК_НАСОСА"
  # "К_ВЕНТИЛЯТОР"
  # "К_ПИТ_РЕГ_Т"
  # "К_ПИТ_РЕГ_УР"
  # "К_УР_ВОДЫ_MIN"
  # "К_УР_ВОДЫ_MAX"
  # "К_ПИТ_НАСОС_ОХЛ"
  # "К_ЛОГ_ВХОД_P_ВбакеКомпрессора"
  # "К_ЛОГ_ВХОД_P_Впатрубке"
  # "К_ЛОГ_ВХОД_T_Врубашке"
  # "К_ЛОГ_ВХОД_T_Вбаке"
  # "К_ЛОГ_ВХОД_P_ВтрубеСидер"
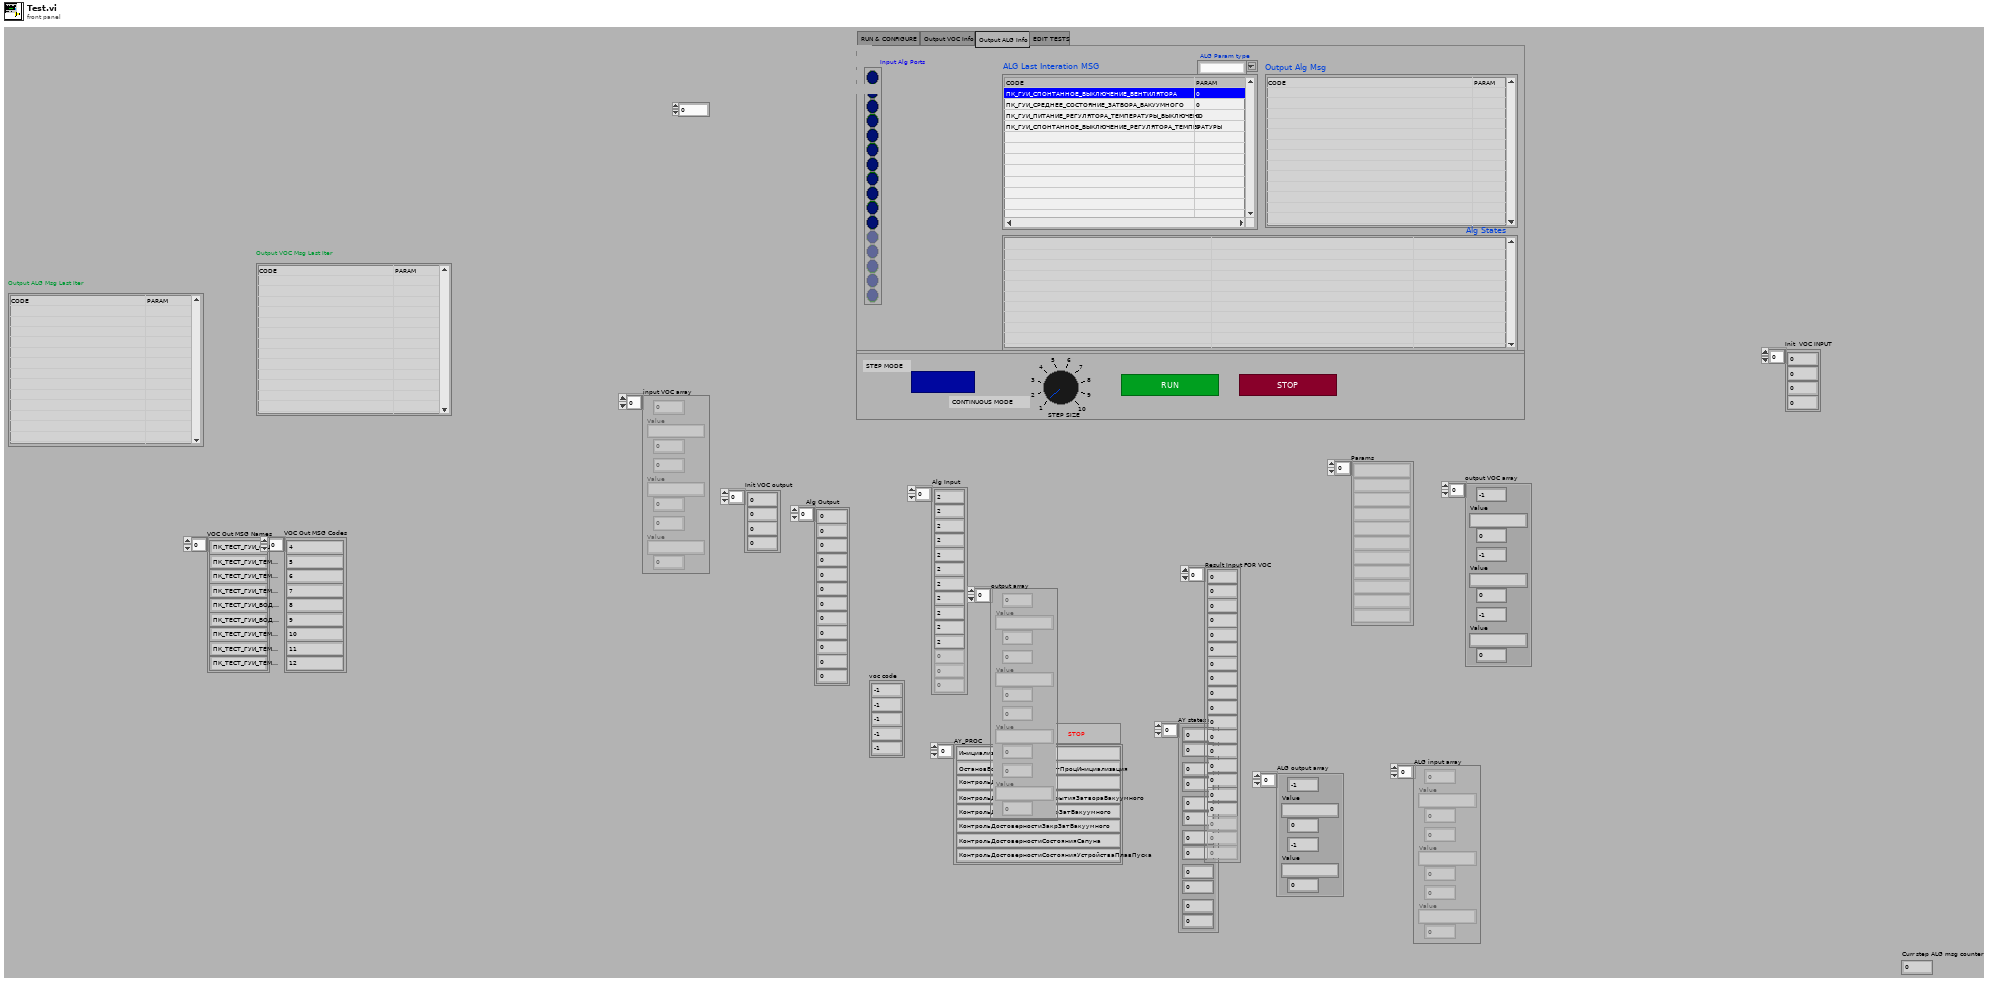
[diagram p1: front panel]
types:
  T1 = enum32{"RUN & CONFIGURE", "Output VOC Info", "Output ALG Info", "EDIT TESTS"}
  T2 = enum16{"open", "open or create", "create or replace", "create", "open (read only)"}
  T3 = cluster{"trimmed string":string, "trimmed string":string}[]
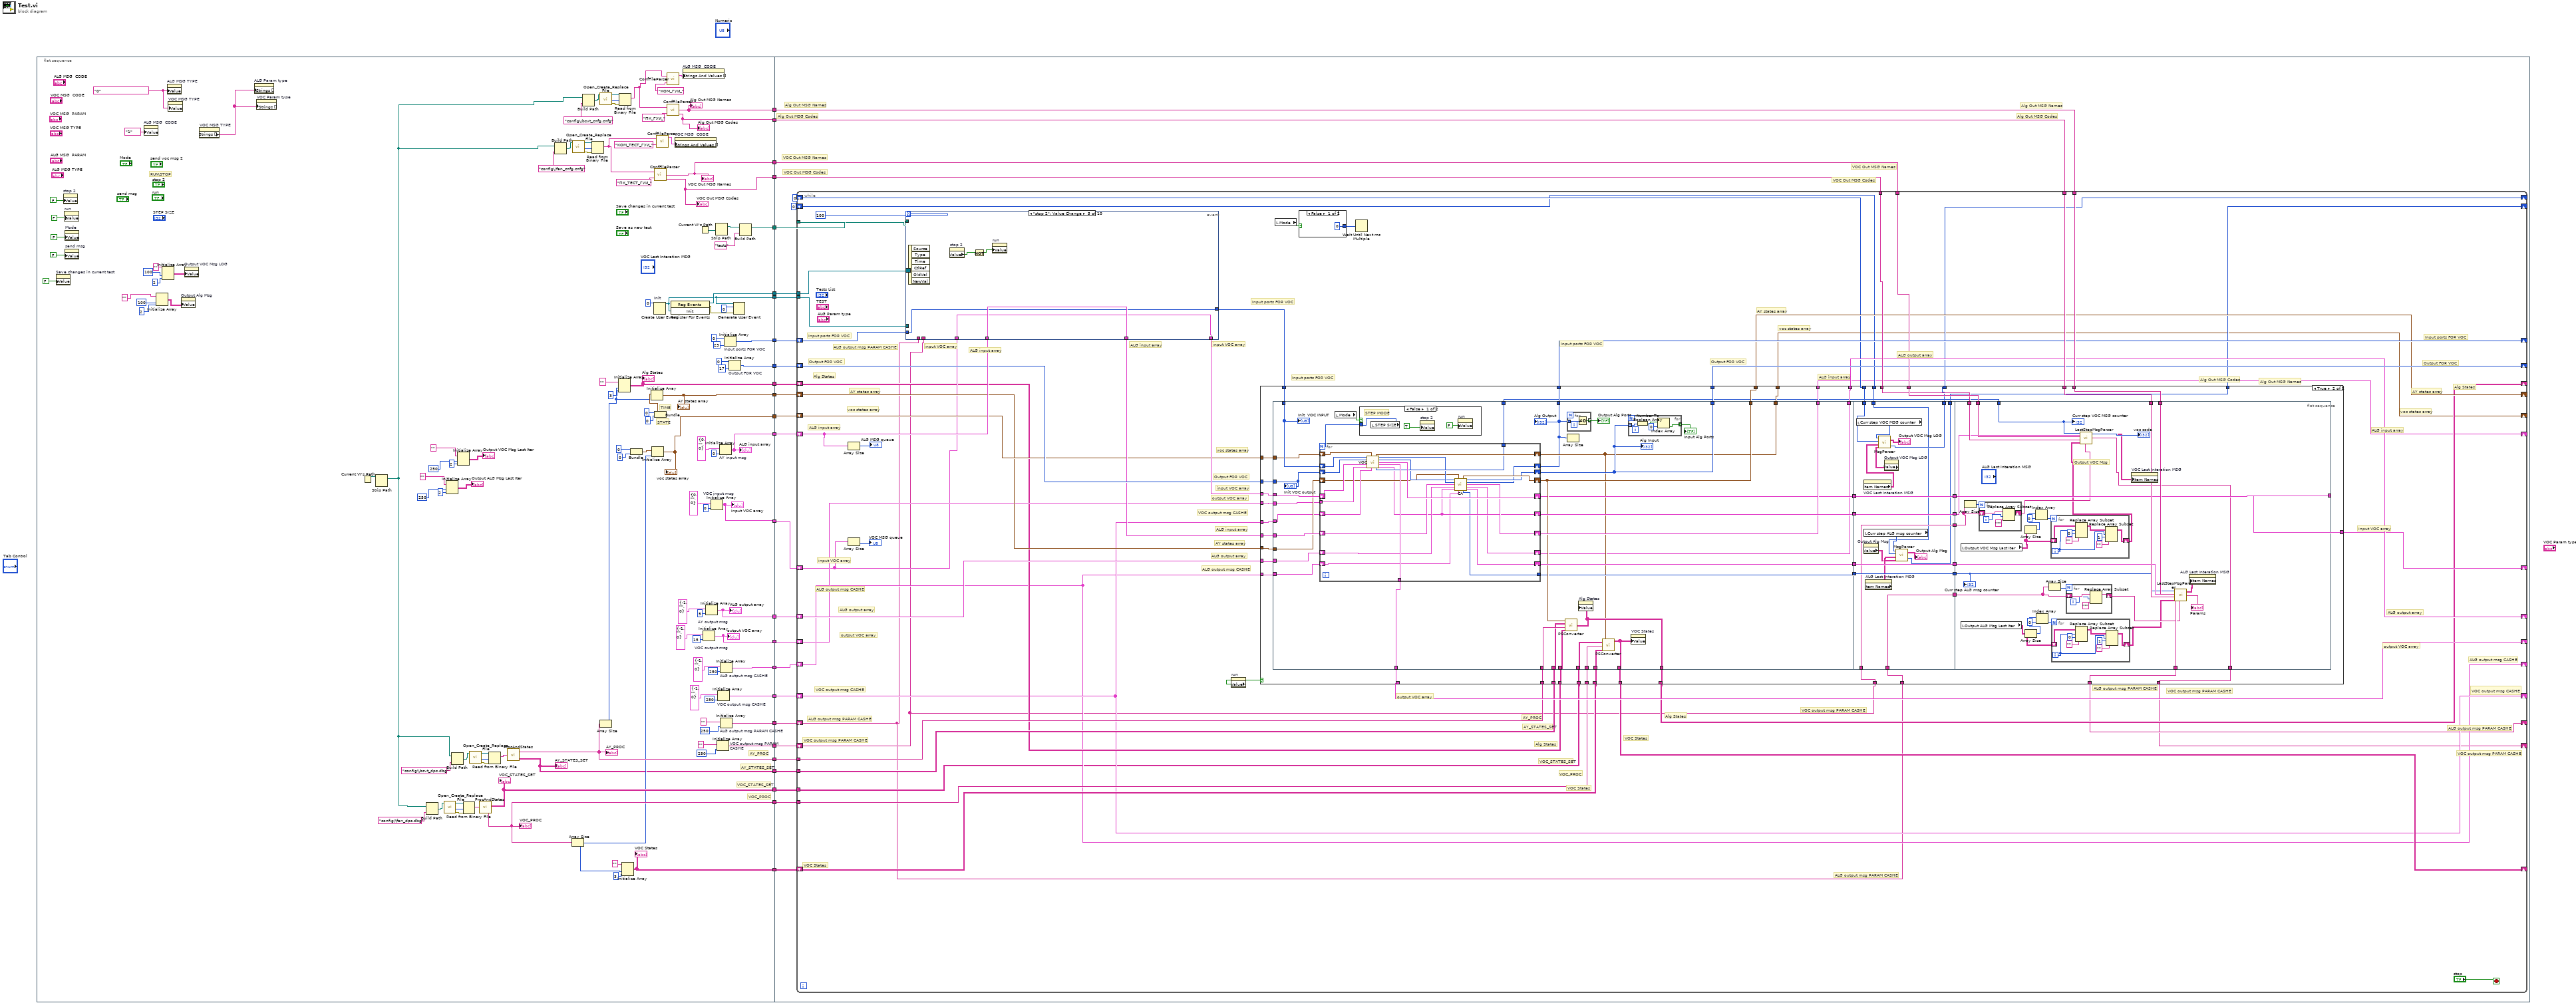
[diagram p0: block diagram]
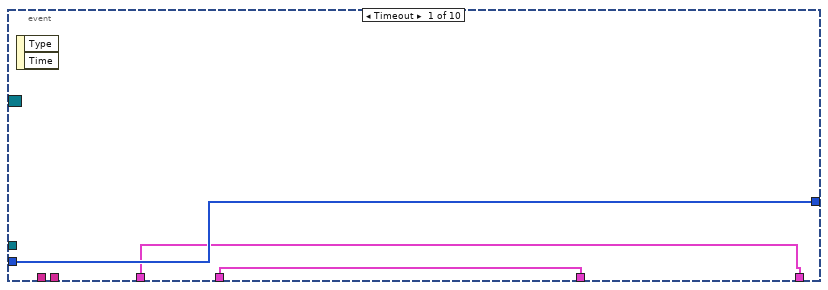
[diagram p2: hidden frame]
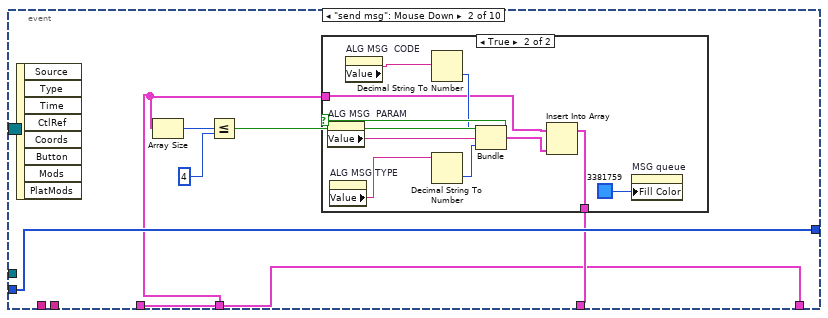
[diagram p3: hidden frame]
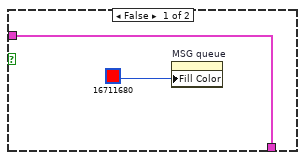
[diagram p4: hidden frame]
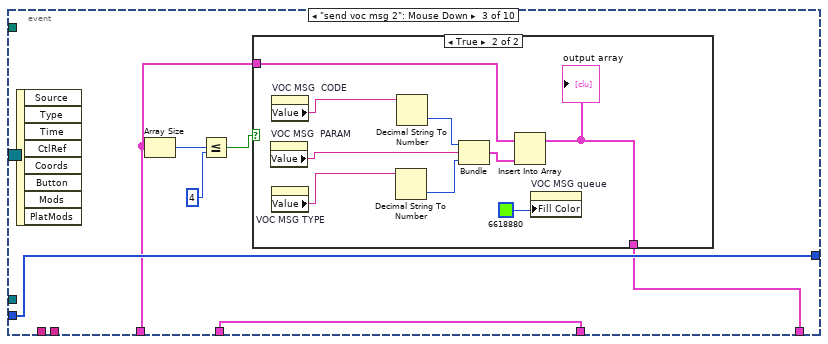
[diagram p5: hidden frame]
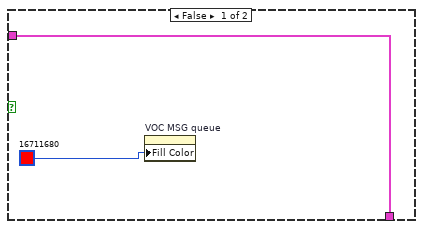
[diagram p6: hidden frame]
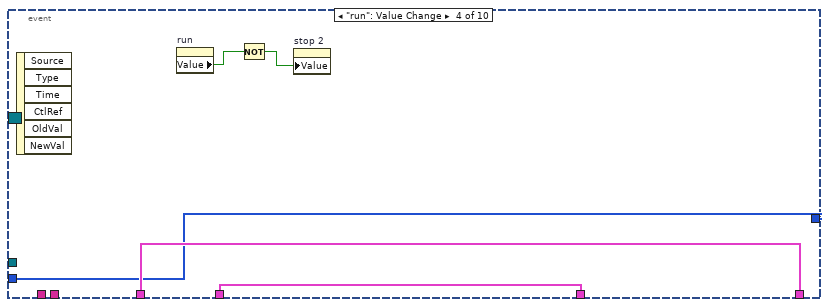
[diagram p7: hidden frame]
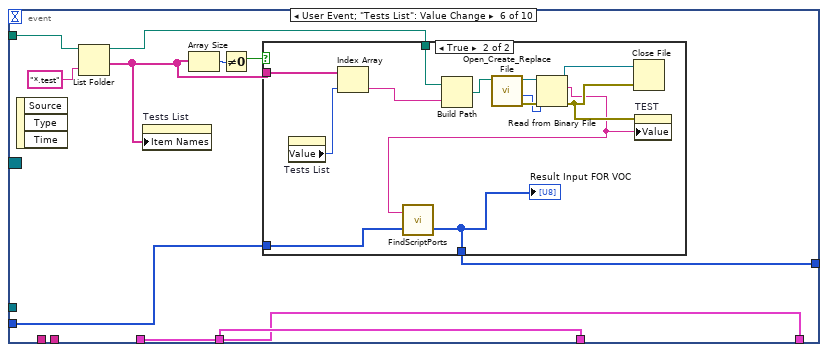
[diagram p8: hidden frame]
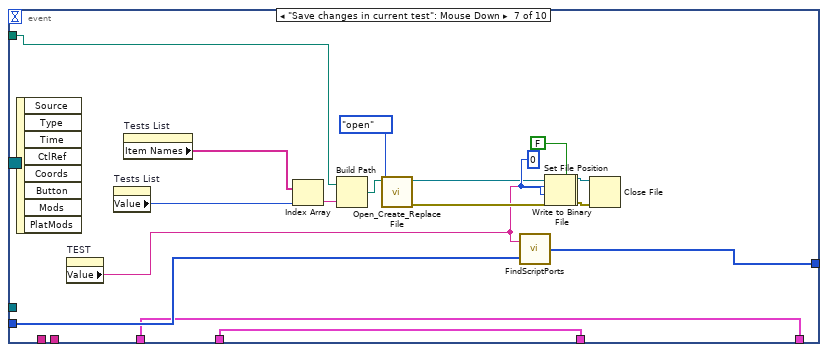
[diagram p10: hidden frame]
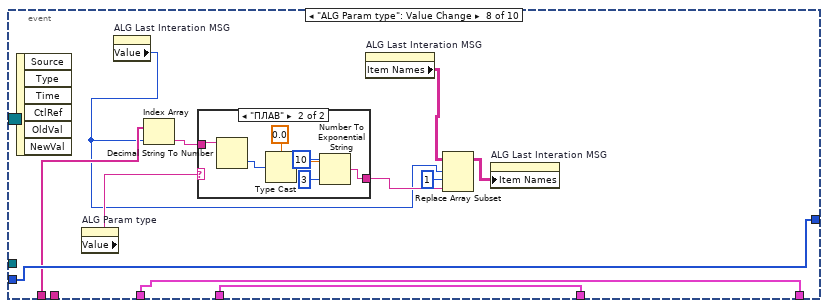
[diagram p11: hidden frame]
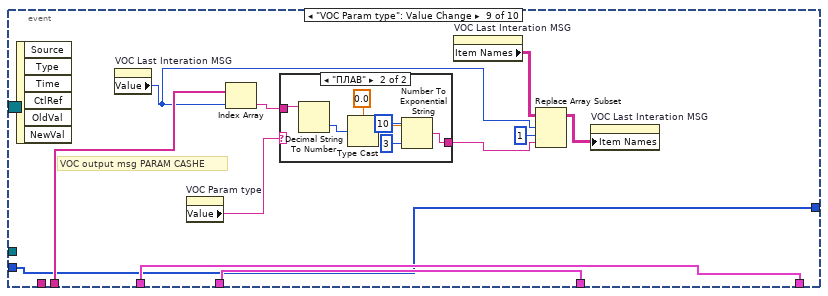
[diagram p13: hidden frame]
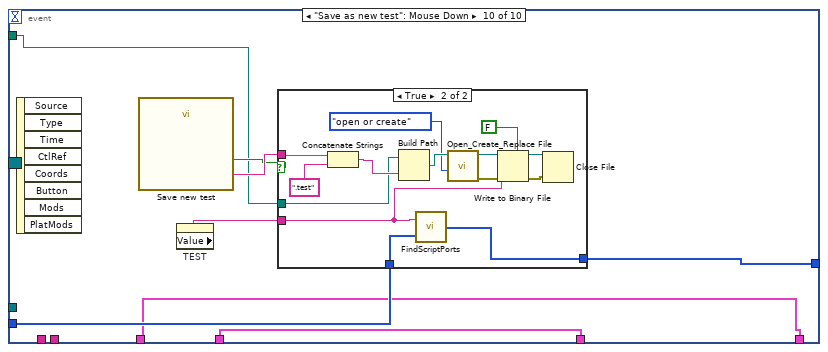
[diagram p15: hidden frame]
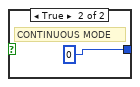
[diagram p17: hidden frame]
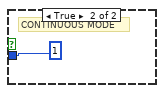
[diagram p19: hidden frame]
diagram:
  n1 = flat-sequence {
    tunnel: [w89] -> w25
    tunnel: [w81] -> w24
    tunnel: [w85] -> w23
    tunnel: [w82] -> w22
    tunnel: [w80] -> w21
    tunnel: [w79] -> w20
    tunnel: [w78] -> w19
    tunnel: [w76] -> w18
    tunnel: [w75] -> w17
    tunnel: [w74] -> w16
    tunnel: [w73] -> w15
    tunnel: [w70] -> w14
    tunnel: [w67] -> w13
    tunnel: [w66] -> w12
    tunnel: [w65] -> w11
    tunnel: [w64] -> w10
    tunnel: [w63] -> w9
    tunnel: [w48] -> w8
    tunnel: [w40] -> w7
    tunnel: [w42] -> w6
    tunnel: [w47] -> w5
    tunnel: [w46] -> w4
    tunnel: [w45] -> w3
    tunnel: [w37] -> w2
    tunnel: [w34] -> w1
    tunnel: w25 -> [w171]
    tunnel: w24 -> [w170]
    tunnel: w23 -> [w169]
    tunnel: w22 -> [w168]
    tunnel: w21 -> [w167]
    tunnel: w20 -> [w166]
    tunnel: w19 -> [w165]
    tunnel: w18 -> [w164]
    tunnel: w17 -> [w163]
    tunnel: w16 -> [w162]
    tunnel: w15 -> [w161]
    tunnel: w14 -> [w160]
    tunnel: w13 -> [w159]
    tunnel: w12 -> [w156]
    tunnel: w11 -> [w155]
    tunnel: w10 -> [w158]
    tunnel: w9 -> [w157]
    tunnel: w8 -> [w153]
    tunnel: w7 -> [w152]
    tunnel: w6 -> [w151]
    tunnel: w5 -> [w150]
    tunnel: w4 -> [w149]
    tunnel: w3 -> [w148]
    tunnel: w2 -> [w146]
    tunnel: w1 -> [w145]
    frame #0 {
      w88 = 0  # Init
      w134 = "0" ("TYPE")
      # "VOC_STATES_SET"
      # "VOC_PROC"
      # "AY_STATES_SET"
      # "AY_PROC"
      # "STATE"
      # "TIME"
      # "RUN\\STOP"
      n2 = property on="Save changes in current test" class="Bool (strict)"("Value"=FALSE ("Save changes in current test")) -> ()  [unwired: 2 in, 2 out]
      n3 = property on="stop 2" class="Bool (strict)"("Value"=FALSE ("send msg 3")) -> ()  [unwired: 2 in, 2 out]
      n4 = property on="run" class="Bool (strict)"("Value"=FALSE ("send msg 2")) -> ()  [unwired: 2 in, 2 out]
      n5 = property on="Mode" class="Bool (strict)"("Value"=FALSE ("Mode")) -> ()  [unwired: 2 in, 2 out]
      n6 = property on="send msg" class="Bool (strict)"("Value"=FALSE ("send msg")) -> ()  [unwired: 2 in, 2 out]
      n7 = property on="ALG MSG  CODE" class="CmbBox"("Value"="1" ("CODE")) -> ()  [unwired: 2 in, 2 out]
      n8 = Initialize Array("" ("element"), 100 ("dimension size"), 2 ("dimension size")) -> (w53:string[][])
      n9 = Initialize Array("" ("element"), 100 ("dimension size"), 2 ("dimension size")) -> (w54:string[][])
      n10 = property on="ALG MSG TYPE" class="CmbBox"("Value"=w134) -> ()  [unwired: 2 in, 2 out]
      n11 = property on="VOC MSG TYPE" class="CmbBox"("Value"=w134) -> ()  [unwired: 2 in, 2 out]
      n12 = property on="Output Alg Msg" class="Tbl (strict)"("Value"=w53) -> ()  [unwired: 2 in, 2 out]
      n13 = property on="Output VOC Msg LOG" class="Tbl (strict)"("Value"=w54) -> ()  [unwired: 2 in, 2 out]
      n14 = property on="VOC MSG TYPE" class="CmbBox"() -> ("Strings []"=w131:string[])  [unwired: 2 in, 2 out]
      n15 = property on="ALG Param type" class="CmbBox"("Strings []"=w131) -> ()  [unwired: 2 in, 2 out]
      n16 = property on="VOC Param type" class="CmbBox"("Strings []"=w131) -> ()  [unwired: 2 in, 2 out]
      n17 = Current VI's Path() -> (path=w62:path)
      n18 = Strip Path(path=w62) -> (stripped path=w61:path)  [unwired: 1 out]
      n19 = Build Path(base path=w61, name or relative path="config\\fan_dps.dbg") -> (appended path=w111:path)
      n20 = call <vilib>:"Open_Create_Replace File.vi"("file path"=w111) -> ("error out"=w110:errorcluster, "file size (bytes)"=w109:i32, "refnum"=w108:refnum<file>)  [unwired: 7 in, 1 out]
      n21 = Initialize Array("" ("Value"), 250 ("dimension size"), 2 ("dimension size")) -> (→"Output ALG Msg Last Iter":string[][])
      n22 = Build Path(base path=w61, name or relative path="config\\bsvt_dps.dbg") -> (appended path=w103:path)
      n23 = Initialize Array("" ("Value"), 250 ("dimension size"), 2 ("dimension size")) -> (→"Output VOC Msg Last Iter":string[][])
      n24 = Read from Binary File(8:w110, 10:w109, 11:w108) -> (2:w77:string)  [unwired: 3 in, 3 out]
      n25 = call <vilib>:"Open_Create_Replace File.vi"("file path"=w103) -> ("error out"=w102:errorcluster, "file size (bytes)"=w101:i32, "refnum"=w100:refnum<file>)  [unwired: 7 in, 1 out]
      n26 = call "ProcAndStates.vi"("spreadsheet string"=w77) -> ("PROCESSES"=w42:string[], "STATES"=w47:string[][])
      "VOC_PROC" <- w42
      "VOC_STATES_SET" <- w47
      n27 = Read from Binary File(8:w102, 10:w101, 11:w100) -> (2:w113:string)  [unwired: 3 in, 3 out]
      n28 = call "ProcAndStates.vi"("spreadsheet string"=w113) -> ("PROCESSES"=w48:string[], "STATES"=w40:string[][])
      "AY_PROC" <- w48
      "AY_STATES_SET" <- w40
      n29 = Build Path(base path=w61, name or relative path="config\\fan_cnfg.cnfg") -> (appended path=w127:path)
      n30 = Array Size(array=w42) -> (size(s)=w41:i32)
      n31 = call <vilib>:"Open_Create_Replace File.vi"("file path"=w127) -> ("error out"=w126:errorcluster, "file size (bytes)"=w125:i32, "refnum"=w124:refnum<file>)  [unwired: 7 in, 1 out]
      n32 = Build Path(base path=w61, name or relative path="config\\bsvt_cnfg.cnfg") -> (appended path=w99:path)
      n33 = Read from Binary File(8:w126, 10:w125, 11:w124) -> (2:w129:string)  [unwired: 3 in, 3 out]
      n34 = Array Size(array=w48) -> (size(s)=w56:i32)
      n35 = call <vilib>:"Open_Create_Replace File.vi"("file path"=w99) -> ("error out"=w98:errorcluster, "file size (bytes)"=w97:i32, "refnum"=w96:refnum<file>)  [unwired: 7 in, 1 out]
      n36 = Initialize Array("" ("Value"), w56, 3 ("dimension size")) -> (w46:string[][])
      "Alg States" <- w46
      n37 = Read from Binary File(8:w98, 10:w97, 11:w96) -> (2:w120:string)  [unwired: 3 in, 3 out]
      n38 = Initialize Array("" ("Value"), w41, 3 ("dimension size")) -> (w45:string[][])
      "VOC States" <- w45
      n39 = Bundle(u32 0, u8 0) -> (w119:cluster{u32, u8})  [unwired: 1 in]
      n40 = Initialize Array(w119, w41) -> (w75:cluster{u32, u8}[])
      "voc states array" <- w75
      n41 = Create User Event(user event datatype=w88) -> (user event=w81:refnum<user-event>)  [unwired: 1 in, 1 out]
      n42 = call "ConfFileParser.vi"("TEXT"=w129, "search string"="ПК_ТЕСТ_ГУИ_") -> ("Names"=w64:string[], "Codes"=w63:string[])  [unwired: 1 out]
      "VOC Out MSG Names" <- w64
      "VOC Out MSG Codes" <- w63
      n43 = Bundle(u32 0, u8 0) -> (w116:cluster{u32, u8})  [unwired: 1 in]
      n44 = Initialize Array(w116, w56) -> (w76:cluster{u32, u8}[])
      "AY states array" <- w76
      n45 = call "ConfFileParser.vi"("TEXT"=w129, "search string"="КОМ_ТЕСТ_ГУИ_") -> ("Cluster Array"=w122:T3)  [unwired: 2 out]
      n46 = call "ConfFileParser.vi"("TEXT"=w120, "search string"="КОМ_ГУИ_") -> ("Cluster Array"=w105:T3)  [unwired: 2 out]
      n47 = call "ConfFileParser.vi"("TEXT"=w120, "search string"="ПК_ГУИ_") -> ("Names"=w66:string[], "Codes"=w65:string[])  [unwired: 1 out]
      "Alg Out MSG Names" <- w66
      "Alg Out MSG Codes" <- w65
      n48 = register-events(w81) -> (reference out=w85:refnum<event-registration>, error out=w87:errorcluster)  [unwired: 2 in]
      n49 = property on="VOC MSG  CODE" class="CmbBox"("Strings And Values []"=w122) -> ()  [unwired: 2 in, 2 out]
      n50 = property on="ALG MSG  CODE" class="CmbBox"("Strings And Values []"=w105) -> ()  [unwired: 2 in, 2 out]
      n51 = Current VI's Path() -> (path=w91:path)
      n52 = Initialize Array "VOC output msg"(cluster{i32, "Value":string, i32} {-1, "Value"="", 0} ("element"), 15 ("dimension size")) -> (w73:cluster{i32, "Value":string, i32}[])
      "output VOC array" <- w73
      n53 = Initialize Array "AY output msg"(cluster{i32, "Value":string, i32} {-1, "Value"="", 0} ("element"), 5 ("dimension size")) -> (w74:cluster{i32, "Value":string, i32}[])
      "ALG output array" <- w74
      n54 = Initialize Array "VOC input msg"(cluster{i32, "Value":string, i32} {0, "Value"="", 0} ("element"), 0 ("dimension size")) -> (w79:cluster{i32, "Value":string, i32}[])
      "input VOC array" <- w79
      n55 = Strip Path(path=w91) -> (stripped path=w90:path)  [unwired: 1 out]
      n56 = Initialize Array "VOC output msg PARAM CASHE"("" ("Value"), 250 ("dimension size")) -> (w34:string[])
      n57 = Initialize Array "VOC output msg CASHE"(cluster{i32, "Value":string, i32} {-1, "Value"="", 0} ("element"), 250 ("dimension size")) -> (w70:cluster{i32, "Value":string, i32}[])
      n58 = Initialize Array "AY input msg"(cluster{i32, "Value":string, i32} {0, "Value"="", 0} ("element"), 0 ("dimension size")) -> (w80:cluster{i32, "Value":string, i32}[])
      "ALG input array" <- w80
      n59 = Initialize Array "ALG output msg PARAM CASHE"("" ("Value"), 250 ("dimension size")) -> (w37:string[])
      n60 = Initialize Array "ALG output msg CASHE"(cluster{i32, "Value":string, i32} {-1, "Value"="", 0} ("element"), 250 ("dimension size")) -> (w67:cluster{i32, "Value":string, i32}[])
      n61 = Initialize Array "Input ports FOR VOC"(u8 0 ("element"), 23 ("dimension size")) -> (w82:u8[])
      n62 = Initialize Array "Output FOR VOC"(u8 0 ("element"), 17 ("dimension size")) -> (w78:u8[])
      n63 = Generate User Event(user event=w81, event data cluster=0, error in=w87) -> ()  [unwired: 2 out]
      n64 = Build Path(base path=w90, name or relative path="tests") -> (appended path=w89:path)
    }
    frame #1 {
      # "VOC Out MSG Names"
      # "Alg Out MSG Codes"
      # "Alg Out MSG Names"
      # "VOC Out MSG Codes"
      # "VOC Out MSG Codes"
      # "VOC Out MSG Names"
      # "Alg Out MSG Codes"
      # "Alg Out MSG Names"
      n65 = while {
        tunnel: w171 -> [w213]
        tunnel: w170 -> [w216]
        tunnel: w169 -> [w217]
        shift-right: [w199] -> _
        shift-left: w168 -> [w215]
        shift-right: [w178] -> _
        shift-left: w167 -> [w212]
        shift-right: [w193] -> _
        shift-left: w166 -> [w196]
        shift-right: [w198] -> _
        shift-left: w165 -> [w209]
        shift-right: [w197] -> _
        shift-left: w164 -> [w206]
        shift-right: [w177] -> _
        shift-left: w163 -> [w207]
        shift-right: [w195] -> _
        shift-left: w162 -> [w205]
        shift-right: [w194] -> _
        shift-left: w161 -> [w204]
        shift-right: [w180] -> _
        shift-left: w160 -> [w180]
        shift-right: [w179] -> _
        shift-left: w159 -> [w179]
        tunnel: w158 -> [w203]
        tunnel: w157 -> [w202]
        tunnel: w156 -> [w200]
        tunnel: w155 -> [w201]
        shift-right: [w190] -> _
        shift-left: 0 -> [w191]
        tunnel: w151 -> [w187]
        tunnel: w153 -> [w189]
        tunnel: w152 -> [w188]
        tunnel: w150 -> [w176]
        shift-right: [w185] -> _
        shift-left: w149 -> [w186]
        shift-right: [w183] -> _
        shift-left: w148 -> [w184]
        shift-right: [w181] -> _
        shift-left: 0 -> [w182]
        shift-right: [w175] -> _
        shift-left: w146 -> [w174]
        shift-right: [w172] -> _
        shift-left: w145 -> [w173]
        stop <- "stop" stop-if-true
        # "VOC output msg PARAM CASHE"
        # "VOC output msg PARAM CASHE"
        # "VOC output msg PARAM CASHE"
        # "VOC output msg PARAM CASHE"
        # "ALG output msg PARAM CASHE"
        # "ALG output msg PARAM CASHE"
        # "ALG output msg PARAM CASHE"
        # "ALG output msg PARAM CASHE"
        # "ALG output msg PARAM CASHE"
        # "voc states array"
        # "VOC States"
        # "Alg States"
        # "VOC States"
        # "VOC States"
        # "Alg States"
        # "Alg States"
        # "Alg States"
        # "VOC_STATES_SET"
        # "VOC_PROC"
        # "AY_STATES_SET"
        # "AY_PROC"
        # "output VOC array"
        # "AY states array"
        # "ALG output array"
        # "ALG input array"
        # "ALG output msg CASHE"
        # "VOC output msg CASHE"
        # "output VOC array"
        # "ALG output array"
        # "input VOC array"
        # "ALG input array"
        # "voc states array"
        # "AY states array"
        # "Output FOR VOC"
        # "Input ports FOR VOC"
        # "Output FOR VOC"
        # "Input ports FOR VOC"
        # "Alg Out MSG Codes"
        # "Alg Out MSG Names"
        # "ALG output msg CASHE"
        # "ALG output msg CASHE"
        # "VOC output msg CASHE"
        # "VOC output msg CASHE"
        # "ALG output array"
        # "output VOC array"
        # "output VOC array"
        # "ALG output array"
        # "AY states array"
        # "voc states array"
        # "voc states array"
        # "AY states array"
        # "ALG input array"
        # "Output FOR VOC"
        # "Output FOR VOC"
        # "input VOC array"
        # "Input ports FOR VOC"
        # "input VOC array"
        # "ALG input array"
        # "input VOC array"
        # "input VOC array"
        # "Input ports FOR VOC"
        # "Input ports FOR VOC"
        # "ALG input array"
        # "ALG input array"
        n66 = Array Size(array=w212) -> (size(s)=→"ALG MSG queue":i32)
        n67 = Array Size(array=w196) -> (size(s)=→"VOC MSG queue":i32)
        n68 = event shown="[4] \"stop 2\": Value Change" {
          selector: w217 -> [_ _ _ _ _ _ _ _ _ _]
          dyn-events: _ -> [_ _ _ _ _ _ _ _ _ _]
          timeout: 100 -> [_ _ _ _ _ _ _ _ _ _]
          tunnel: w215 -> [w225 w232 w249 w262 w267 w279 w310 w323 w334 w358]
          tunnel: w216 -> [_ _ _ _ _ _ _ _ _ _]
          tunnel: [w225 w232 w249 w262 w267 w278 w309 w323 w334 w357] -> w211
          tunnel: w213 -> [_ _ _ _ _ w275 w308 _ _ w356]
          tunnel: w212 -> [w224 w228 w250 w264 w269 w273 w306 w325 w336 w355]
          tunnel: [w224 w227 w250 w264 w269 w273 w306 w325 w336 w355] -> w208
          tunnel: w196 -> [w223 w226 w245 w263 w268 w272 w305 w324 w335 w354]
          tunnel: [w223 w226 w244 w263 w268 w272 w305 w324 w335 w354] -> w210
          tunnel: w174 -> [_ _ _ _ _ _ _ w318 _ _]
          tunnel: w173 -> [_ _ _ _ _ _ _ _ w343 _]
          event Timeout {
            n69 = event-data() -> ()  [unwired: 1 in, 2 out]
          }
          event "send msg": Mouse Down {
            n70 = event-data() -> ()  [unwired: 1 in, 8 out]
            n71 = Array Size(array=w228) -> (size(s)=w231:i32)
            n72 = Less Or Equal?(x=w231, y=4) -> (x <= y?=w229:bool)
            n73 = case shown="True" w229 {
              tunnel: w228 -> [w233 w237]
              tunnel: [w233 w235] -> w227
              frame False {
                n74 = property on="MSG queue" class="Slide (strict)"("Fill Color"=u32 16711680) -> ()  [unwired: 2 in, 2 out]
              }
              frame True {
                n75 = property on="ALG MSG  PARAM" class="Str"() -> ("Value"=w242:string)  [unwired: 2 in, 2 out]
                n76 = property on="ALG MSG TYPE" class="CmbBox"() -> ("Value"=w240:string)  [unwired: 2 in, 2 out]
                n77 = property on="ALG MSG  CODE" class="CmbBox"() -> ("Value"=w239:string)  [unwired: 2 in, 2 out]
                n78 = Decimal String To Number(string=w239) -> (number=w241:i32)  [unwired: 2 in, 1 out]
                n79 = Decimal String To Number(string=w240) -> (number=w243:i32)  [unwired: 2 in, 1 out]
                n80 = Bundle(w241, "Value"=w242, w243) -> (w236:cluster{i32, "Value":string, i32})  [unwired: 1 in]
                n81 = Insert Into Array(array=w237, new element=w236) -> (w235:cluster{i32, "Value":string, i32}[])  [unwired: 1 in]
                n82 = property on="MSG queue" class="Slide (strict)"("Fill Color"=u32 3381759) -> ()  [unwired: 2 in, 2 out]
              }
            }
          }
          event "send voc msg 2": Mouse Down {
            n83 = event-data() -> ()  [unwired: 1 in, 8 out]
            n84 = Array Size(array=w245) -> (size(s)=w246:i32)
            n85 = Less Or Equal?(x=w246, y=4) -> (x <= y?=w248:bool)
            n86 = case shown="True" w248 {
              tunnel: w245 -> [w251 w259]
              tunnel: [w251 w253] -> w244
              frame False {
                n87 = property on="VOC MSG queue" class="Slide (strict)"("Fill Color"=u32 16711680) -> ()  [unwired: 2 in, 2 out]
              }
              frame True {
                n88 = property on="VOC MSG  PARAM" class="Str"() -> ("Value"=w257:string)  [unwired: 2 in, 2 out]
                n89 = property on="VOC MSG  CODE" class="CmbBox"() -> ("Value"=w258:string)  [unwired: 2 in, 2 out]
                n90 = property on="VOC MSG TYPE" class="CmbBox"() -> ("Value"=w256:string)  [unwired: 2 in, 2 out]
                n91 = Decimal String To Number(string=w256) -> (number=w261:i32)  [unwired: 2 in, 1 out]
                n92 = Decimal String To Number(string=w258) -> (number=w260:i32)  [unwired: 2 in, 1 out]
                n93 = Bundle(w260, "Value"=w257, w261) -> (w254:cluster{i32, "Value":string, i32})  [unwired: 1 in]
                n94 = Insert Into Array(array=w259, new element=w254) -> (w253:cluster{i32, "Value":string, i32}[])  [unwired: 1 in]
                "output array" <- w253
                n95 = property on="VOC MSG queue" class="Slide (strict)"("Fill Color"=u32 6618880) -> ()  [unwired: 2 in, 2 out]
              }
            }
          }
          event "run": Value Change {
            n96 = event-data() -> ()  [unwired: 1 in, 6 out]
            n97 = property on="run" class="Bool (strict)"() -> ("Value"=w266:bool)  [unwired: 2 in, 2 out]
            n98 = Not(x=w266) -> (.not. x?=w265:bool)
            n99 = property on="stop 2" class="Bool (strict)"("Value"=w265) -> ()  [unwired: 2 in, 2 out]
          }
          event "stop 2": Value Change {
            n100 = event-data() -> ()  [unwired: 1 in, 6 out]
            n101 = property on="stop 2" class="Bool (strict)"() -> ("Value"=w271:bool)  [unwired: 2 in, 2 out]
            n102 = Not(x=w271) -> (.not. x?=w270:bool)
            n103 = property on="run" class="Bool (strict)"("Value"=w270) -> ()  [unwired: 2 in, 2 out]
          }
          event User Event; "Tests List": Value Change {
            n104 = event-data() -> ()  [unwired: 1 in, 3 out]
            n105 = List Folder(path=w275, pattern="*.test") -> (path out=w276:path, filenames=w274:string[])  [unwired: 2 in, 2 out]
            n106 = property on="Tests List" class="LstBox (strict)"("Item Names"=w274) -> ()  [unwired: 2 in, 2 out]
            n107 = Array Size(array=w274) -> (size(s)=w281:i32)
            n108 = Not Equal To 0?(x=w281) -> (x != 0?=w280:bool)
            n109 = case shown="True" w280 {
              tunnel: w274 -> [_ w295]
              tunnel: w276 -> [_ w293]
              tunnel: w279 -> [w282 w285]
              tunnel: [w282 w284] -> w278
              frame False {
              }
              frame True {
                n110 = property on="Tests List" class="LstBox (strict)"() -> ("Value"=w283:i32)  [unwired: 2 in, 2 out]
                n111 = Index Array(array=w295, index=w283) -> (element=w294:string)
                n112 = Build Path(base path=w293, name or relative path=w294) -> (appended path=w292:path)
                n113 = call <vilib>:"Open_Create_Replace File.vi"("file path"=w292) -> ("error out"=w290:errorcluster, "file size (bytes)"=w289:i32, "refnum"=w291:refnum<file>)  [unwired: 7 in, 1 out]
                n114 = Read from Binary File(8:w290, 10:w289, 11:w291) -> (0:w287:errorcluster, 2:w286:string, 3:w288:refnum<file>)  [unwired: 3 in, 1 out]
                n115 = call "FindScriptPorts.vi"("Input FOR VOC"=w285, "Test"=w286) -> ("Result Input FOR VOC"=w284:u8[])
                "Result Input FOR VOC" <- w284
                n116 = Close File(refnum=w288, error in=w287) -> ()  [unwired: 2 out]
                n117 = property on="TEST" class="Str"(error in=w287, "Value"=w286) -> ()  [unwired: 1 in, 2 out]
              }
            }
          }
          event "Save changes in current test": Mouse Down {
            w302 = 0 ("pos offset (0)")
            n118 = event-data() -> ()  [unwired: 1 in, 8 out]
            n119 = property on="TEST" class="Str"() -> ("Value"=w299:string)  [unwired: 2 in, 2 out]
            n120 = property on="Tests List" class="LstBox (strict)"() -> ("Value"=w304:i32)  [unwired: 2 in, 2 out]
            n121 = property on="Tests List" class="LstBox (strict)"() -> ("Item Names"=w307:string[])  [unwired: 2 in, 2 out]
            n122 = Index Array(array=w307, index=w304) -> (element=w314:string)
            n123 = Build Path(base path=w308, name or relative path=w314) -> (appended path=w313:path)
            n124 = call <vilib>:"Open_Create_Replace File.vi"("function (open:0)"=T2."open", "file path"=w313) -> ("error out"=w300:errorcluster, "refnum"=w301:refnum<file>)  [unwired: 6 in, 2 out]
            n125 = call "FindScriptPorts.vi"("Input FOR VOC"=w310, "Test"=w299) -> ("Result Input FOR VOC"=w309:u8[])
            n126 = Set File Position(offset (in bytes) (0)=w302, refnum=w301, from (0:start)=w302, error in=w300) -> (refnum out=w298:refnum<file>, error out=w297:errorcluster)
            n127 = Write to Binary File(file (use dialog)=w298, data=w299, error in=w297, 5:FALSE ("prepend array or string size? (T)")) -> (refnum out=w312:refnum<file>, error out=w311:errorcluster)  [unwired: 2 in, 1 out]
            n128 = Close File(refnum=w312, error in=w311) -> ()  [unwired: 2 out]
          }
          event "ALG Param type": Value Change {
            n129 = event-data() -> ()  [unwired: 1 in, 6 out]
            n130 = property on="ALG Param type" class="CmbBox"() -> ("Value"=w319:string)  [unwired: 2 in, 2 out]
            n131 = property on="ALG Last Interation MSG" class="MCListbox (strict)"() -> ("Value"=w315:i32)  [unwired: 2 in, 2 out]
            n132 = Index Array(array=w318, index=w315) -> (element=w322:string)
            n133 = case shown="\"ПЛАВ\"" w319 {
              tunnel: w322 -> [w326 w331]
              tunnel: [w326 w329] -> w321
              frame "False", Default {
              }
              frame "ПЛАВ" {
                n134 = Decimal String To Number(string=w331) -> (number=w333:i32)  [unwired: 2 in, 1 out]
                n135 = Type Cast(type=sgl 0.0, x=w333) -> (*(type *) &x=w330:sgl)
                n136 = Number To Exponential String(number=w330, precision (6)=i16 3, 3:i16 10 ("width (-)")) -> (E-format string=w329:string)  [unwired: 1 in]
              }
            }
            n137 = property on="ALG Last Interation MSG" class="MCListbox (strict)"() -> ("Item Names"=w317:string[][])  [unwired: 2 in, 2 out]
            n138 = Replace Array Subset(array=w317, new element=w321, index (row)=w315, index (col)=1 ("disabled index (col)")) -> (w316:string[][])
            n139 = property on="ALG Last Interation MSG" class="MCListbox (strict)"("Item Names"=w316) -> ()  [unwired: 2 in, 2 out]
          }
          event "VOC Param type": Value Change {
            # "VOC output msg PARAM CASHE"
            n140 = event-data() -> ()  [unwired: 1 in, 6 out]
            n141 = property on="VOC Last Interation MSG" class="MCListbox (strict)"() -> ("Value"=w340:i32)  [unwired: 2 in, 2 out]
            n142 = property on="VOC Param type" class="CmbBox"() -> ("Value"=w342:string)  [unwired: 2 in, 2 out]
            n143 = Index Array(array=w343, index=w340) -> (element=w344:string)
            n144 = case shown="\"ПЛАВ\"" w342 {
              tunnel: w344 -> [w345 w350]
              tunnel: [w345 w348] -> w339
              frame "False", Default {
              }
              frame "ПЛАВ" {
                n145 = Decimal String To Number(string=w350) -> (number=w352:i32)  [unwired: 2 in, 1 out]
                n146 = Type Cast(type=sgl 0.0, x=w352) -> (*(type *) &x=w349:sgl)
                n147 = Number To Exponential String(number=w349, precision (6)=i16 3, 3:i16 10 ("width (-)")) -> (E-format string=w348:string)  [unwired: 1 in]
              }
            }
            n148 = property on="VOC Last Interation MSG" class="MCListbox (strict)"() -> ("Item Names"=w338:string[][])  [unwired: 2 in, 2 out]
            n149 = Replace Array Subset(array=w338, new element=w339, index (row)=w340, index (col)=1 ("disabled index (col)")) -> (w337:string[][])
            n150 = property on="VOC Last Interation MSG" class="MCListbox (strict)"("Item Names"=w337) -> ()  [unwired: 2 in, 2 out]
          }
          event "Save as new test": Mouse Down {
            n151 = event-data() -> ()  [unwired: 1 in, 8 out]
            n152 = call "Save new test"() -> ("Test name"=w360:string, "OK"=w359:bool)  [unwired: 17 in, 1 out]
            n153 = property on="TEST" class="Str"() -> ("Value"=w353:string)  [unwired: 2 in, 2 out]
            n154 = case shown="True" w359 {
              tunnel: w356 -> [_ w367]
              tunnel: w360 -> [_ w374]
              tunnel: w353 -> [_ w365]
              tunnel: w358 -> [w361 w364]
              tunnel: [w361 w363] -> w357
              frame False {
              }
              frame True {
                n155 = Concatenate Strings(w374, ".test" ("string")) -> (w368:string)
                n156 = Build Path(base path=w367, name or relative path=w368) -> (appended path=w369:path)
                n157 = call "FindScriptPorts.vi"("Input FOR VOC"=w364, "Test"=w365) -> ("Result Input FOR VOC"=w363:u8[])
                n158 = call <vilib>:"Open_Create_Replace File.vi"("function (open:0)"=T2."open or create", "file path"=w369) -> ("error out"=w373:errorcluster, "refnum"=w370:refnum<file>)  [unwired: 6 in, 2 out]
                n159 = Write to Binary File(file (use dialog)=w370, data=w365, error in=w373, 5:FALSE ("prepend array or string size? (T)")) -> (refnum out=w371:refnum<file>, error out=w372:errorcluster)  [unwired: 2 in, 1 out]
                n160 = Close File(refnum=w371, error in=w372) -> ()  [unwired: 2 out]
              }
            }
          }
        }
        n161 = property on="run" class="Bool (strict)"() -> ("Value"=w192:bool)  [unwired: 2 in, 2 out]
        n162 = case shown="True" w192 {
          tunnel: w211 -> [w391 w440]
          tunnel: w210 -> [w385 w439]
          tunnel: w209 -> [w390 w438]
          tunnel: w208 -> [w387 w437]
          tunnel: w207 -> [w388 w436]
          tunnel: w206 -> [w389 w435]
          tunnel: w205 -> [w386 w434]
          tunnel: w204 -> [w384 w433]
          tunnel: w180 -> [_ w432]
          tunnel: w179 -> [_ w411]
          tunnel: w203 -> [_ w431]
          tunnel: w202 -> [_ w430]
          tunnel: w201 -> [_ w429]
          tunnel: w200 -> [_ w428]
          tunnel: [w391 w427] -> w199
          tunnel: [w390 w426] -> w198
          tunnel: [w389 w425] -> w197
          tunnel: [w388 w424] -> w177
          tunnel: [w387 w423] -> w178
          tunnel: [w386 w422] -> w195
          tunnel: [w384 w421] -> w194
          tunnel: [w385 w408] -> w193
          tunnel: w191 -> [w383 w395]
          tunnel: [w383 w394] -> w190
          tunnel: w189 -> [_ w419]
          tunnel: w188 -> [_ w418]
          tunnel: w187 -> [_ w417]
          tunnel: w176 -> [_ w416]
          tunnel: w186 -> [w382 w415]
          tunnel: [w382 w414] -> w185
          tunnel: w184 -> [w381 w413]
          tunnel: [w381 w412] -> w183
          tunnel: w182 -> [w380 w393]
          tunnel: [w380 w392] -> w181
          tunnel: w174 -> [w379 w397]
          tunnel: [w379 w410] -> w175
          tunnel: w173 -> [w378 w399]
          tunnel: [w378 w409] -> w172
          frame False {
          }
          frame True {
            n163 = flat-sequence {
              tunnel: w440 -> [w470]
              tunnel: w439 -> [w471]
              tunnel: w438 -> [w447]
              tunnel: w437 -> [w469]
              tunnel: w436 -> [w468]
              tunnel: w435 -> [w467]
              tunnel: w434 -> [w464]
              tunnel: w433 -> [w466]
              tunnel: w432 -> [w465]
              tunnel: w411 -> [w463]
              tunnel: [w462] -> w407
              tunnel: [w461] -> w405
              tunnel: [w442] -> w427
              tunnel: [w446] -> w426
              tunnel: [w459] -> w425
              tunnel: [w445] -> w424
              tunnel: [w460] -> w423
              tunnel: [w444] -> w422
              tunnel: [w458] -> w421
              tunnel: [w457] -> w403
              tunnel: [w456] -> w420
              tunnel: w419 -> [w455]
              tunnel: w418 -> [w443]
              tunnel: w417 -> [w454]
              tunnel: w416 -> [w453]
              tunnel: w415 -> [w452]
              tunnel: [w451] -> w414
              tunnel: w413 -> [w450]
              tunnel: [w449] -> w412
              tunnel: [w448] -> w401
              tunnel: w407 -> [w526]
              tunnel: [w526] -> w406
              tunnel: w405 -> [w525]
              tunnel: [w525] -> w404
              tunnel: w403 -> [w524]
              tunnel: [w524] -> w402
              tunnel: w401 -> [w523]
              tunnel: [w523] -> w400
              tunnel: w399 -> [w522]
              tunnel: [w522] -> w398
              tunnel: w397 -> [w521]
              tunnel: [w521] -> w396
              tunnel: w395 -> [w518]
              tunnel: [w517] -> w394
              tunnel: w393 -> [w510]
              tunnel: [w509] -> w392
              tunnel: [w551] -> w408
              tunnel: w406 -> [w549]
              tunnel: w431 -> [w550]
              tunnel: w430 -> [w555]
              tunnel: w429 -> [w554]
              tunnel: w428 -> [w553]
              tunnel: w404 -> [w552]
              tunnel: w402 -> [w551]
              tunnel: w420 -> [w548]
              tunnel: w400 -> [w542]
              tunnel: [w546] -> w410
              tunnel: [w539] -> w409
              tunnel: w398 -> [w538]
              tunnel: w396 -> [w537]
              frame #0 {
                n164 = local read "Mode"() -> (w474:bool)
                n165 = case shown="False" w474 {
                  tunnel: [w481 1] -> w473
                  frame False {
                    # "STEP MODE"
                    n166 = local read "STEP SIZE"() -> (w481:i32)
                    n167 = property on="stop 2" class="Bool (strict)"("Value"=TRUE ("stop")) -> ()  [unwired: 2 in, 2 out]
                    n168 = property on="run" class="Bool (strict)"("Value"=FALSE ("run")) -> ()  [unwired: 2 in, 2 out]
                  }
                  frame True {
                    # "CONTINUOUS MODE"
                  }
                }
                n169 = for {
                  N: w473 -> [_]
                  shift-right: [w489] -> w442
                  shift-left: w470 -> [w508]
                  shift-right: [w490] -> w446
                  shift-left: w447 -> [w507]
                  shift-right: [w492] -> w460
                  shift-left: w469 -> [w496]
                  shift-right: [w502] -> w445
                  shift-left: w468 -> [w503]
                  shift-right: [w488] -> w444
                  shift-left: w464 -> [w495]
                  shift-right: [w493] -> w459
                  shift-left: w467 -> [w494]
                  shift-right: [w500] -> w457
                  shift-left: w471 -> [w505]
                  tunnel: w466 -> [w504]
                  shift-right: [w491] -> w462
                  shift-left: w465 -> [w506]
                  shift-right: [w486] -> w461
                  shift-left: w463 -> [w487]
                  tunnel: [w501] -> w458
                  tunnel: [w499] -> w456
                  tunnel: [w485] -> w448
                  n170 = call "VOC.vi"("input VOC ports"=w508, "voc states array"=w503, "output VOC ports"=w507, "Input VOC msg Array"=w505, "output VOC msg array"=w504, "VOC output msg CASHE"=w506) -> ("Filled voc states array"=w502:cluster{u32, u8}[], "Modified input VOC ports"=w498:u8[], "Modified output VOC ports"=w497:u8[], "Clear Input VOC msg Array"=w500:cluster{i32, "Value":string, i32}[], "clear output VOC array"=w501:cluster{i32, "Value":string, i32}[], "Curr step output MSG counter"=w499:i32, "Filled VOC output msg CASHE"=w491:cluster{i32, "Value":string, i32}[])  [unwired: 3 in]
                  n171 = call "CA.vi"("init input ports"=w497, "Alg states"=w494, "output"=w498, "input ALG msg array"=w496, "Output ALG msg array"=w495, "VOC output msg CASHE"=w491, "ALG output msg CASHE"=w487) -> ("Output Alg states"=w493:cluster{u32, u8}[], "input ports"=w490:u8[], "modified output ports"=w489:i8[], "Clear ALG input array"=w492:cluster{i32, "Value":string, i32}[], "Clear ALG output array"=w488:cluster{i32, "Value":string, i32}[], "Curr step msg counter"=w485:i32, "Modified ALG output msg CASHE"=w486:cluster{i32, "Value":string, i32}[])  [unwired: 2 in]
                }
                "Alg Input" <- w446
                "Alg Output" <- w442
                n172 = call "PSConverter.vi"("Current States 2"=w452, "PROC"=w455, "STATES"=w443, "Input claster"=w459) -> ("Current States"=w451:string[][])
                n173 = for {
                  tunnel: w442 -> [w480] mode=indexing
                  tunnel: [w479] -> w472 mode=indexing
                  n174 = Not Equal To 0?(x=w480) -> (x != 0?=w479:bool)
                }
                "Output Alg Ports" <- w472
                n175 = Array Size(array=w442) -> ()  [unwired: 1 out]
                n176 = property on="Alg States" class="Tbl (strict)"("Value"=w451) -> ()  [unwired: 2 in, 2 out]
                n177 = call "PSConverter.vi"("Current States 2"=w450, "PROC"=w454, "STATES"=w453, "Input claster"=w445) -> ("Current States"=w449:string[][])
                n178 = for {
                  tunnel: w446 -> [w478] mode=indexing
                  tunnel: [w476] -> w441 mode=indexing
                  n179 = Number To Boolean Array(number=w478) -> (Boolean array=w477:bool[])
                  n180 = Index Array(array=w477, index=0) -> (element=w476:bool)
                }
                "Input Alg Ports" <- w441
                n181 = property on="VOC States" class="Tbl (strict)"("Value"=w449) -> ()  [unwired: 2 in, 2 out]
                "Init  VOC INPUT" <- w470
                "Init VOC output" <- w447
              }
              frame #1 {
                n182 = local read "Curr step VOC MSG counter"() -> (w520:i32)
                n183 = local read "Curr step ALG msg counter"() -> (w511:i32)
                n184 = property on="VOC Last Interation MSG" class="MCListbox (strict)"() -> ("Item Names"=w513:string[][])  [unwired: 2 in, 2 out]
                n185 = property on="Output Alg Msg" class="Tbl (strict)"() -> ("Value"=w512:string[][])  [unwired: 2 in, 2 out]
                n186 = property on="ALG Last Interation MSG" class="MCListbox (strict)"() -> ("Item Names"=w515:string[][])  [unwired: 2 in, 2 out]
                n187 = property on="Output VOC Msg LOG" class="Tbl (strict)"() -> ("Value"=w514:string[][])  [unwired: 2 in, 2 out]
                n188 = call "MsgParser.vi"("Result Output Msg Table"=w514, "Output VOC Msg LOG"=w513, "MSG Counter"=w518, "current msg num"=w520) -> ("Result Counter"=w517:i32, "Output Alg Msg"=→"Output VOC Msg LOG":string[][])
                n189 = call "MsgParser.vi"("Result Output Msg Table"=w512, "Output VOC Msg LOG"=w515, "MSG Counter"=w510, "current msg num"=w511) -> ("Result Counter"=w509:i32, "Output Alg Msg"=→"Output Alg Msg":string[][])
              }
              frame #2 {
                # "Output VOC Msg"
                n190 = local read "Output VOC Msg Last Iter"() -> (w536:string[][])
                n191 = local read "Output ALG Msg Last Iter"() -> (w528:string[][])
                n192 = Array Size(array=w538) -> (size(s)=w541:i32)
                n193 = for {
                  N: w541 -> [_]
                  shift-right: [w573] -> w540
                  shift-left: w538 -> [w575]
                  i -> [w574]
                  n194 = Replace Array Subset(array=w575, new element="*" ("new element/subarray"), index=w574) -> (w573:string[])
                }
                n195 = Array Size(array=w536) -> (size(s)=w535:i32[])
                n196 = Array Size(array=w528) -> (size(s)=w531:i32[])
                n197 = Index Array(array=w535, index=0) -> (element=w533:i32)
                n198 = Index Array(array=w531, index=0) -> (element=w529:i32)
                n199 = Array Size(array=w537) -> (size(s)=w545:i32)
                n200 = for {
                  N: w533 -> [_]
                  shift-right: [w565] -> w532
                  shift-left: w536 -> [w572]
                  i -> [w566]
                  n201 = Replace Array Subset(array=w572, new element="" ("new element/subarray"), index (row)=w566, index (col)=0 ("disabled index (col)")) -> (w567:string[][])
                  n202 = Replace Array Subset(array=w567, new element="" ("new element/subarray"), index (row)=w566, index (col)=1 ("disabled index (col)")) -> (w565:string[][])
                }
                n203 = for {
                  N: w529 -> [_]
                  shift-right: [w557] -> w527
                  shift-left: w528 -> [w564]
                  i -> [w558]
                  n204 = Replace Array Subset(array=w564, new element="" ("new element/subarray"), index (row)=w558, index (col)=0 ("disabled index (col)")) -> (w559:string[][])
                  n205 = Replace Array Subset(array=w559, new element="" ("new element/subarray"), index (row)=w558, index (col)=1 ("disabled index (col)")) -> (w557:string[][])
                }
                n206 = for {
                  N: w545 -> [_]
                  shift-right: [w577] -> w543
                  shift-left: w537 -> [w579]
                  i -> [w578]
                  n207 = Replace Array Subset(array=w579, new element="*" ("new element/subarray"), index=w578) -> (w577:string[])
                }
                n208 = call "LastStepMsgParser.vi"("Params array"=w540, "Output Msg Table"=w532, "Out MSG Codes"=w555, "output msg array"=w549, "Out MSG Names"=w550, "current msg num"=w548) -> ("Params"=w539:string[], "code"=→"voc code":i32[], "Output Alg Msg"=w547:string[][])  [unwired: 2 in]
                n209 = property on="VOC Last Interation MSG" class="MCListbox (strict)"("Item Names"=w547) -> ()  [unwired: 2 in, 2 out]
                n210 = call "LastStepMsgParser.vi"("Params array"=w543, "Output Msg Table"=w527, "Out MSG Codes"=w554, "output msg array"=w552, "Out MSG Names"=w553, "current msg num"=w542) -> ("Params"=w546:string[], "Output Alg Msg"=w544:string[][])  [unwired: 2 in, 1 out]
                "Params" <- w546
                n211 = property on="ALG Last Interation MSG" class="MCListbox (strict)"("Item Names"=w544) -> ()  [unwired: 2 in, 2 out]
                "Curr step VOC MSG counter" <- w548
                "Curr step ALG msg counter" <- w542
              }
            }
          }
        }
        n212 = local read "Mode"() -> (w220:bool)
        n213 = case shown="False" w220 {
          tunnel: [u32 0 ("millisecond multiple") u32 0 ("millisecond multiple")] -> w219
          frame False {
          }
          frame True {
            # "CONTINUOUS MODE"
          }
        }
        n214 = Wait Until Next ms Multiple(millisecond multiple=w219) -> ()  [unwired: 1 out]
      }
    }
  }
